vi "Q14070-Z060B - 副本.vi"() -> ()   [LabVIEW 2013]
uses:
  <vilib>/Utility/file.llb/Read From Spreadsheet File (string).vi
  <vilib>/express/express arith-compare/Formula/XNode/ExpressFormulaBlockNode.xnode
  PCI8622_32.dll
  <vilib>/printing/EasyPrintingControls.llb/contents.ctl
  <vilib>/Utility/NIReport.llb/NI_ReportGenerationCore.lvlib
  <vilib>/printing/EasyPrintingControls.llb/report_type.ctl
  <vilib>/printing/EasyPrinting.llb/Easy Print VI Panel or Documentation (path).vi
  <vilib>/Utility/NIReport.llb/NI_report.lvclass
panel:
  in  "确定按钮":bool
  out "员工ID":string
  in  "出支线工步号":dbl
  out "报警提示":string
  in  "报警工步号":dbl
  out "急停":bool
  in  "机械间隙值":dbl
  out "DeviceHandle":u32
  in  "轴向力设定次数":dbl=5.0
  in  "最小间隙(mm)":dbl=0.0005 format="%#.3f"
  out "本备料状态H":bool
  out "本测试状态H":bool
  out "本自动状态H":bool
  out "夹头松开":bool
  out "测头右位":bool
  out "测头左位":bool
  in  "测头气缸右移":bool
  in  "测头气缸左移":bool
  in  "轴向力已做次数":dbl
  out "轴向力及全行程间隙合格":bool
  out "轴向力启动":bool
  out "间隙启动":bool
  out "夹头夹紧位":bool
  in  "夹头松开":bool
  in  "夹头夹紧":bool
  out "找帽扭矩":dbl=1.0 caption="压力传感器" format="%#.2f"
  out "error out":errorcluster
  out "型号数量":i32
  out "error out 4":errorcluster
  in  "间隙设定调整次数":dbl=5.0
  out "读取产品ID":string
  out "本备料状态":bool
  out "本测试状态":bool
  out "本自动状态":bool
  out "FGCS":string
  out "KSJJ":string
  out "Z060BRFID":string
  out "轴向力Y":dbl[](array[numeric])
  out "轴向力X":dbl[](array[numeric])
  out "间隙X数组":dbl[](array[numeric])
  out "间隙Y数组":dbl[](array[numeric])
  out "error out 3":errorcluster caption="错误输出"
  out "rfid工步号":u32
  out "芯片ID":string="201209190001"
  out "rfid完成":bool
  out "rfid触发":bool
  out "本序已做":bool
  in  "回零完成":bool
  in  "电动缸回零":bool
  in  "单点间隙已调试次数":dbl
  in  "需调整角度(度)":dbl
  out "转向器中心":dbl
  out "扭矩到达":bool
  out "黄灯":bool
  out "红灯":bool
  out "基准位移":dbl caption="压力传感器" format="%#.4f"
  out "上序不合格":bool
  out "单点间隙合格":bool
  out "上序合格":bool
  out "测头机构电机":u32
  out "复位":bool
  in  "型号选择":u16(ring)=1 items=["J709", "J728", "J706"]
  in  "联线按钮":bool
  in  "工步号":u32
  in  "产品ID":string="201209190001"
  out "间隙位移(mm)":dbl caption="压力传感器" format="%#.3f"
  out "齿条推拉力(N)":dbl format="%#.2f"
  out "齿条扭矩(Nm)":dbl format="%#.2f"
  out "通讯状态":bool
  in  "员工ID":string
  out "员工姓名":string
  out "工步提示":string
  out "ADODB._Connection Out 2":refnum<k7>
  out "旋转齿条电机":u32
  out "电动缸电机":u32
  in  "停止":bool
  in  "参数加载":bool
  in  "选项卡控件":T1(tab)
  in  "180°外全行程间隙标准(mm)":dbl=0.1 format="%#.3f"
  out "扭动曲线":cluster{"Y":dbl[], "Y":dbl[]}[](graph) caption="压球涨堵头1"
  out "中间位置间隙":dbl caption="间隙值L(mm)" format="%#.3f"
  in  "中间位置最大间隙标准(mm)":dbl=0.07 format="%#.3f"
  out "右180°外全行程间隙":dbl caption="正向最大间隙L1(mm)" format="%#.3f"
  out "左180°外全行程间隙":dbl caption="正向最大间隙L1(mm)" format="%#.3f"
  out "右180°内全行程间隙":dbl caption="正向最大间隙L1(mm)" format="%#.3f"
  out "左180°内全行程间隙":dbl caption="正向最大间隙L1(mm)" format="%#.3f"
  in  "180°内全行程间隙标准(mm)":dbl=0.07 format="%#.3f"
  in  "找帽OK":bool
  out "左全行程间隙":dbl caption="正向最大间隙L1(mm)" format="%#.3f"
  out "右全行程间隙":dbl caption="正向最大间隙L1(mm)" format="%#.3f"
  out "总圈数最大值":dbl
  out "总圈数标准":dbl
  out "总行程最大值":dbl
  out "总行程标准(mm)":dbl
  out "力波动标准(N)":dbl=60.0 caption="L+Lmax(mm)" format="%#.3f"
  out "最大轴向力标准(N)":dbl=200.0 caption="L+Lmax(mm)" format="%#.3f"
  out "平均轴向力标准(N)":dbl=100.0 caption="L+Lmax(mm)" format="%#.3f"
  out "右轴向力波动(N)":dbl caption="L+Lmax(mm)" format="%#.3f"
  out "右最大轴向力(N)":dbl caption="L+Lmax(mm)" format="%#.3f"
  out "左轴向力波动(N)":dbl caption="最大位移偏离Lmax(mm)" format="%#.3f"
  out "左最大轴向力(N)":dbl caption="最大位移偏离Lmax(mm)" format="%#.3f"
  out "行程跳动曲线":cluster{"Y":dbl[], "Y":dbl[]}[](graph) caption="压球涨堵头1"
  out "右平均轴向力(N)":dbl caption="L+Lmax(mm)" format="%#.3f"
  out "左平均轴向力(N)":dbl caption="最大位移偏离Lmax(mm)" format="%#.3f"
  out "平均轴向力标准(N) max":dbl=200.0 caption="L+Lmax(mm)" format="%#.3f"
  out "总行程":dbl
  out "总圈数":dbl format="%#.2f"
  in  "不合格品":bool
  in  "扭矩停止值":dbl=16.0
  in  "齿条右极限":dbl=-70.0 caption="压力传感器" format="%#.2f"
  in  "齿条左极限":dbl=-262.0 caption="压力传感器" format="%#.2f"
  in  "齿条移动速度":dbl=5.0 caption="压力传感器" format="%#.2f"
  in  "旋转齿条轴找帽转速":dbl=5.0 caption="压力传感器" format="%#.2f"
  in  "测量点扭矩":dbl=4.0 caption="压力传感器" format="%#.2f"
  in  "旋转齿条轴测量转速":dbl caption="压力传感器" format="%#.2f"
  in  "测头机构轴后退位":dbl=30.0 caption="压力传感器" format="%#.2f"
  in  "测头机构轴待检位":dbl caption="压力传感器" format="%#.2f"
  in  "测头机构轴检测位":dbl caption="压力传感器" format="%#.2f"
  in  "测头机构轴移动速度":dbl caption="压力传感器" format="%#.2f"
  in  "全行程修正":dbl=5.5
  in  "夹头松开":bool
  in  "夹头夹紧":bool
  in  "测头气缸右移":bool
  in  "测头气缸左移":bool
  in  "支线下降":bool
  in  "支线顶升":bool
  in  "出支线":bool
  in  "进支线":bool
  in  "主线下降":bool
  in  "主线顶升":bool
  in  "下阻挡器放行":bool
  in  "上阻挡器放行":bool
  in  "测头机构轴使能":bool
  in  "测头机构轴后退":bool
  in  "测头机构轴前进":bool
  in  "电动缸速度(mm/s)":dbl=10.0 format="%#.3f"
  out "电动缸位置(mm)":dbl=10000.0 format="%#.3f"
  in  "旋转齿条轴速度(°/s)":dbl=10.0 format="%#.3f"
  out "旋转齿条轴位置(°)":dbl=10000.0 format="%#.3f"
  in  "测头机构轴速度(mm/s)":dbl=10.0 format="%#.3f"
  out "测头机构轴位置(mm)":dbl=10000.0 format="%#.3f"
  in  "旋转齿条轴右转":bool
  in  "旋转齿条轴左转":bool
  in  "旋转齿条轴使能":bool
  in  "电动缸后退":bool
  in  "电动缸使能":bool
  in  "电动缸前进":bool
  in  "齿条扭矩比例偏移":dbl=1.0 format="%#.2f"
  in  "齿条扭矩零点偏移":dbl format="%#.2f"
  in  "齿条推拉力比例偏移":dbl=1.0 format="%#.2f"
  in  "齿条推拉力零点偏移":dbl format="%#.2f"
  in  "间隙位移比例偏移":dbl=1.0 format="%#.2f"
  in  "间隙位移零点偏移":dbl format="%#.2f"
  in  "传感器参数保存":bool
  in  "参数修改":bool
  in  "参数查询":bool
  in  "参数浏览表":string[][](table)
  # "芜湖机械转向器装配线"
  # "间隙及轴向力检测"
  # "Q14070机械转向器装配线"
  # "湖北唯思凌科装备制造有限公司 设计开发 (C)2015"
  # "间隙测量结果"
  # "间隙测量判定值"
  # "≤"
  # "≤"
  # "≤"
  # "轴向力测量结果"
  # "轴向力测量标准"
  # "≥"
  # "≤"
  # "≥"
  # "≤"
  # "≤"
  # "≥"
  # "不得大于20NM"
  # "传感器校验区"
  # "关于传感器校验：\n1、传感器校验需要由具备资质的单位或部门进行校验。\n2、具备权限的用户才能够修改传感器校验参数和试验参数。\n3、修改校验参数方法：先将比例偏移置为1，修改零点偏移，使零点值与校验的传感器一致；然后根据增幅调整比例偏移。"
  # "注意：\n具备权限的用户才能够修改传感器校验参数和试验参数！"
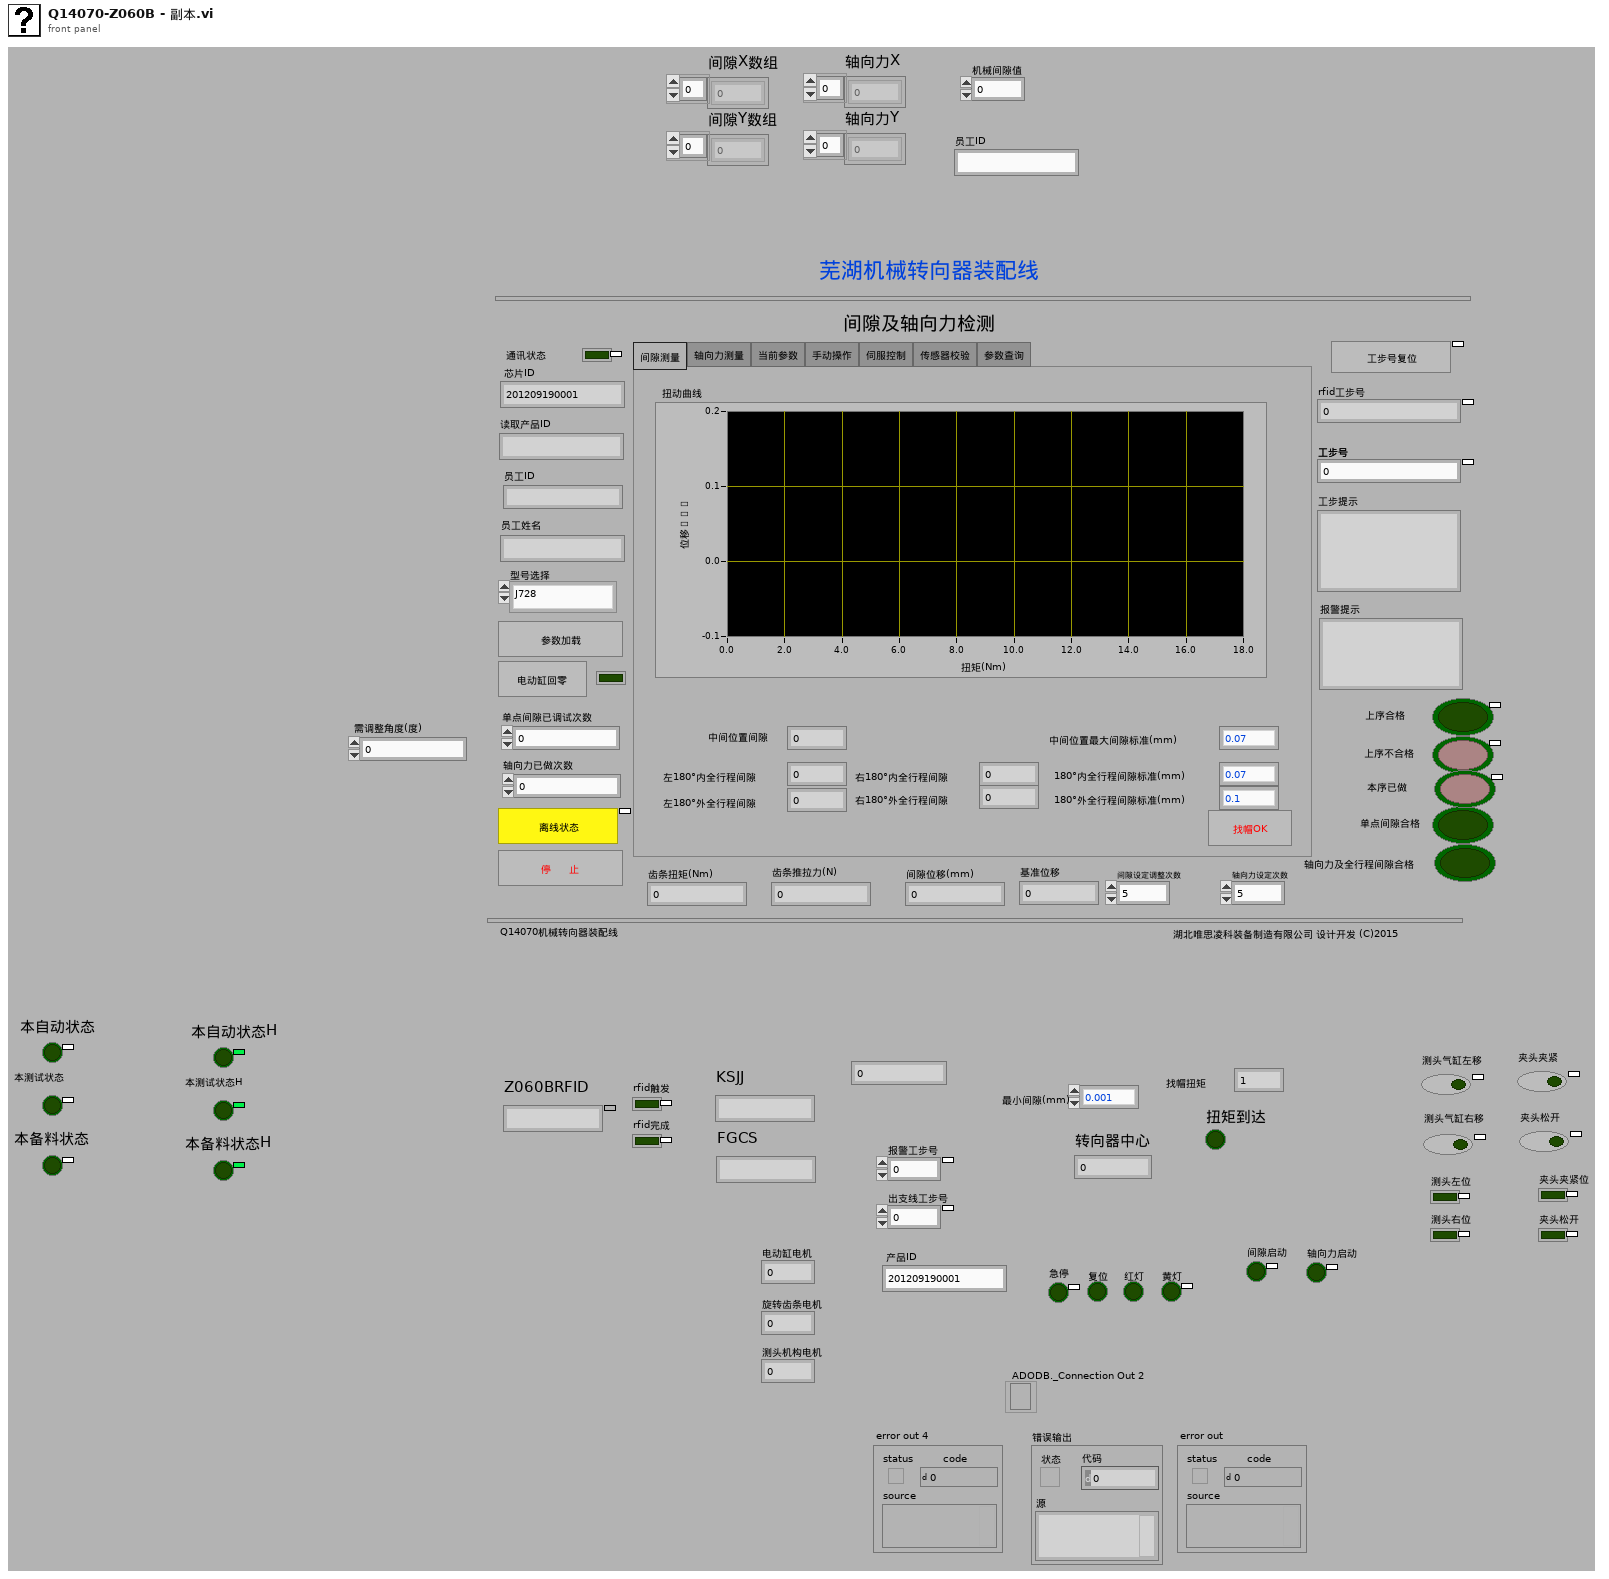
[diagram p1: front panel]
types:
  T1 = enum32{"间隙测量", "轴向力测量", "当前参数", "手动操作", "伺服控制", "传感器校验", "参数查询"}
  T2 = typedef "NI_ReportGenerationCore.lvlib/report_type.ctl" = u16
  T3 = typedef "NI_ReportGenerationCore.lvlib/contents.ctl" = u16
  T4 = typedef "imagedata.ctl" = cluster{"image type":i32, "image depth":i32, "image":u8[], "mask":u8[], "colors":u32[], "Rectangle":cluster{"left":i16, "top":i16, "right":i16, "bottom":i16}}
  T5 = enum8{"Enabled", "Disabled", "Disabled and Grayed Out"}
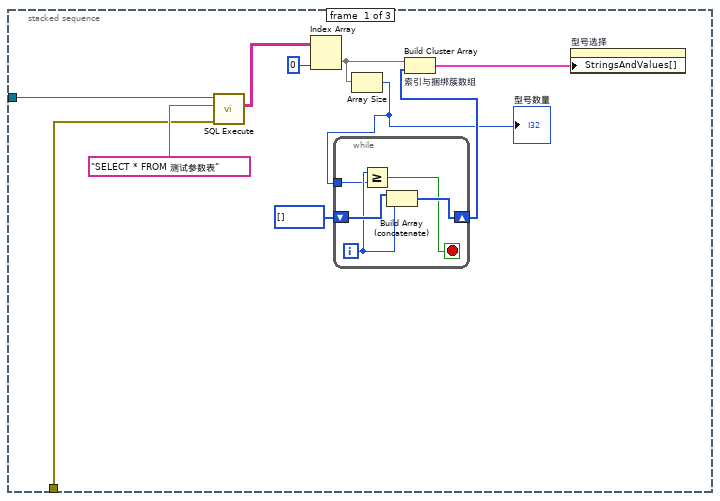
[diagram p4: hidden frame]
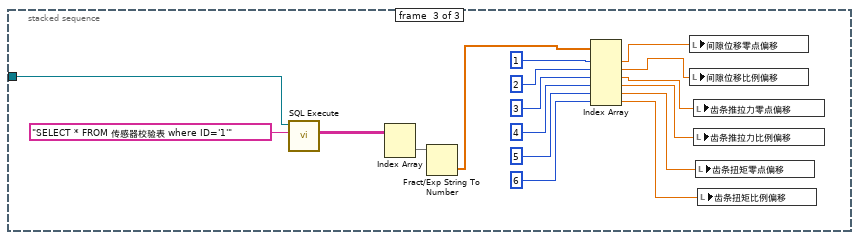
[diagram p5: hidden frame]
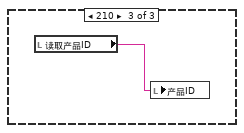
[diagram p7: hidden frame]
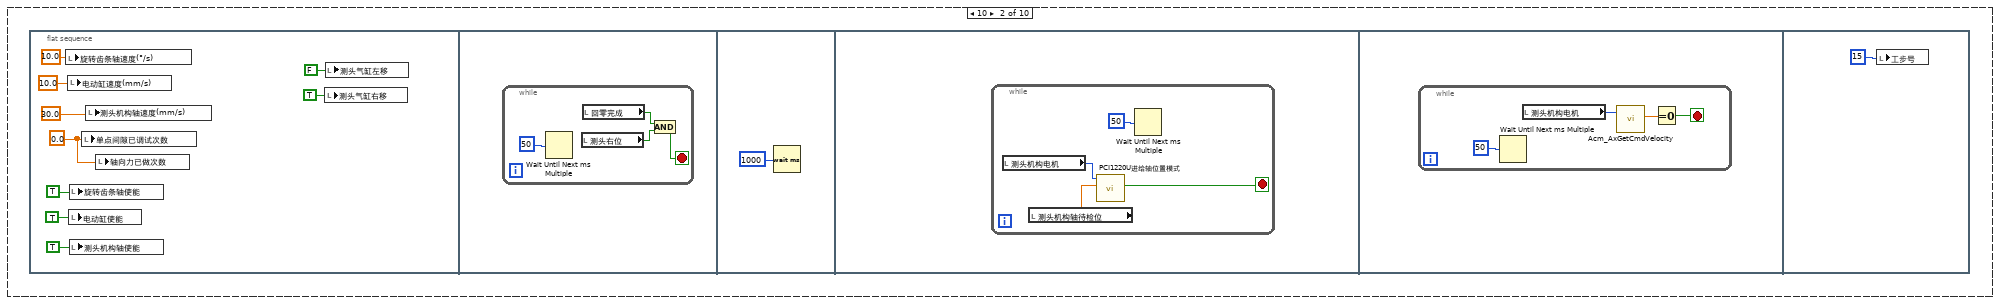
[diagram p9: hidden frame]
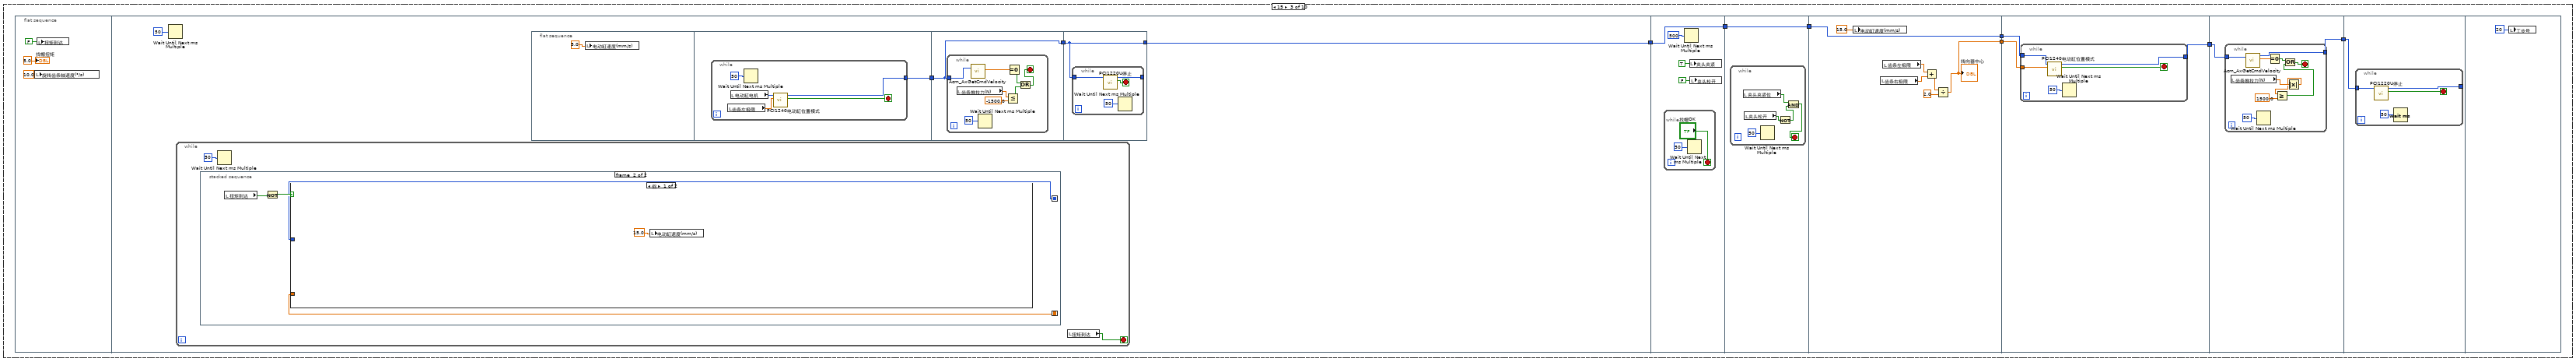
[diagram p10: hidden frame]
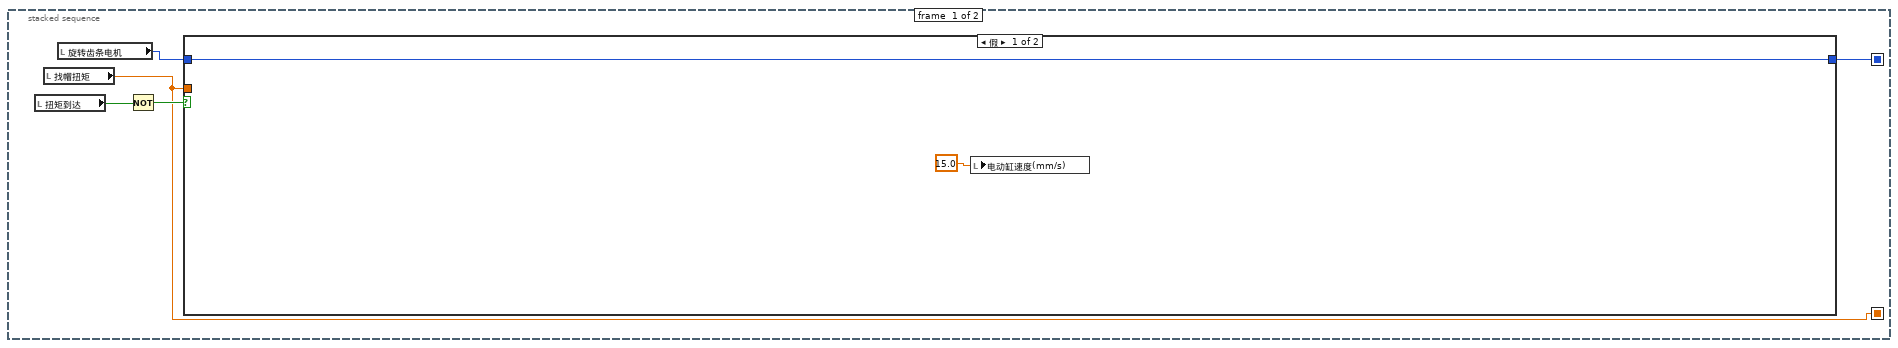
[diagram p11: hidden frame]
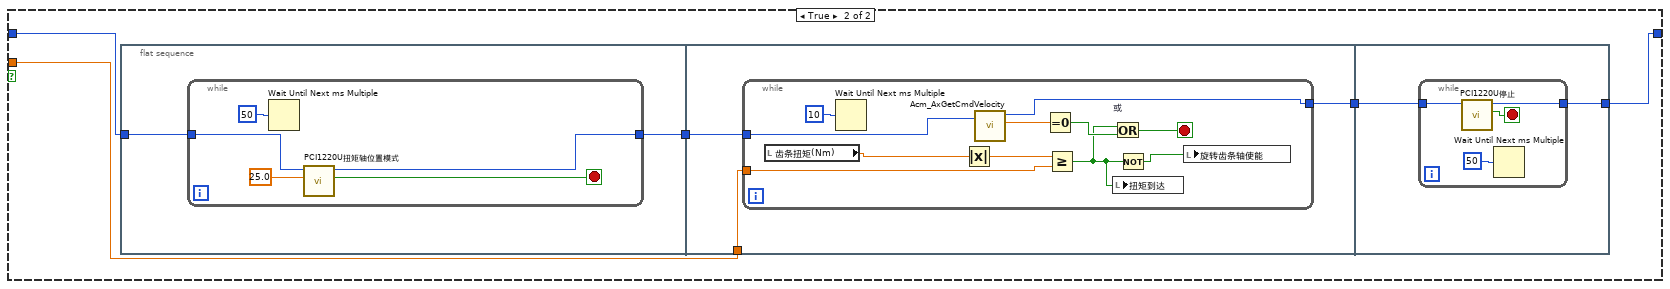
[diagram p12: hidden frame]
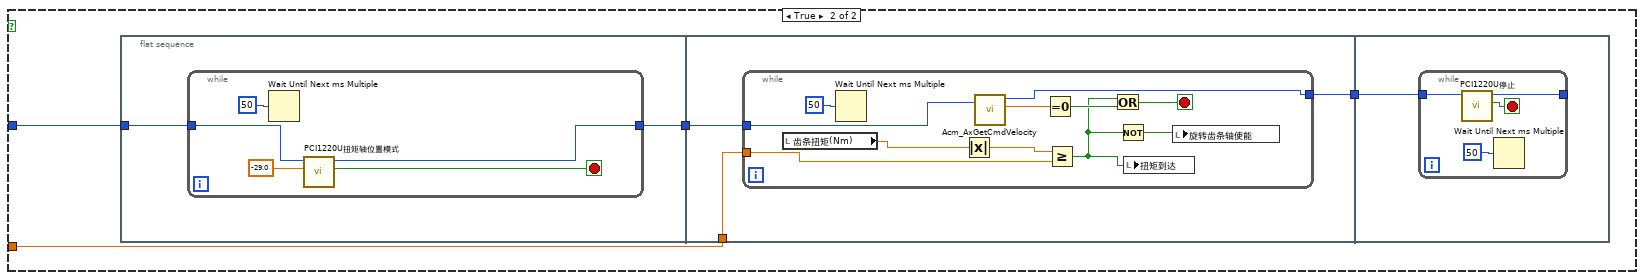
[diagram p13: hidden frame]
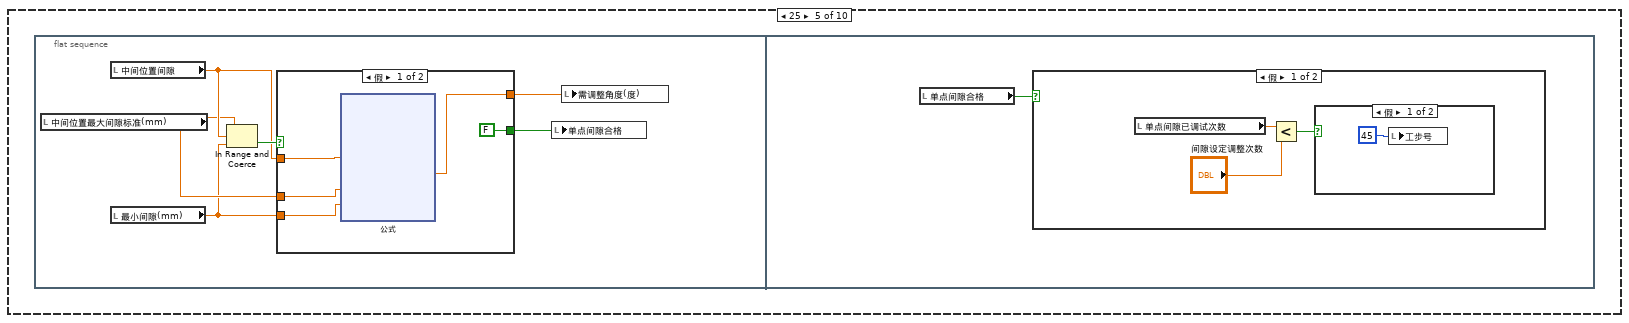
[diagram p15: hidden frame]
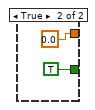
[diagram p16: hidden frame]
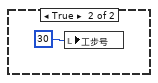
[diagram p17: hidden frame]
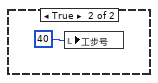
[diagram p18: hidden frame]
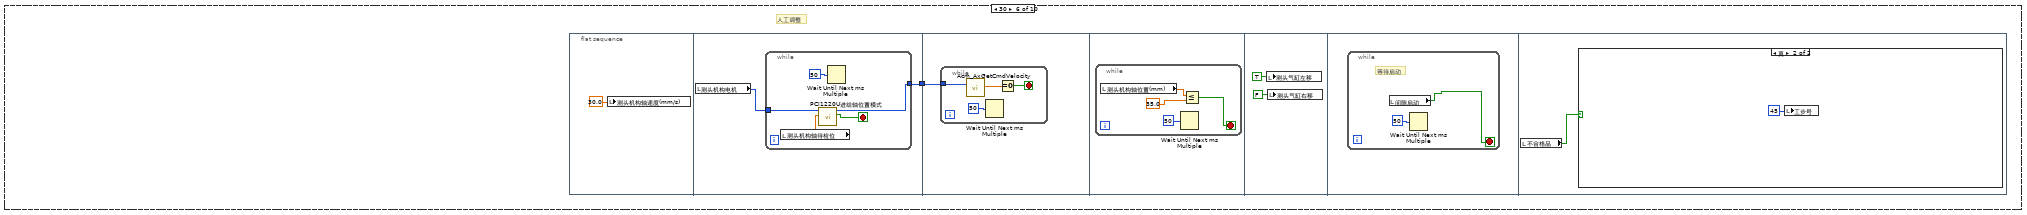
[diagram p19: hidden frame]
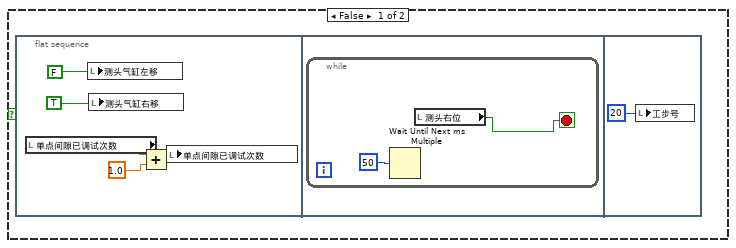
[diagram p20: hidden frame]
diagram:
  n1 = while {
    stop <- w7 stop-if-true
    n2 = local read "工步号"() -> (w5:u32)
    n3 = case shown="20" w5 {
      frame 0, Default {
      }
      frame 10 {
        n4 = flat-sequence {
          frame #0 {
            w8 = 0.0 ("已调试次数")
            n5 = local write "旋转齿条轴速度(°/s)"(10.0 ("旋转齿条轴速度(°/s)")) -> ()
            n6 = local write "电动缸速度(mm/s)"(10.0 ("电动缸速度(mm/s)")) -> ()
            n7 = local write "电动缸使能"(TRUE ("电动缸使能")) -> ()
            n8 = local write "旋转齿条轴使能"(TRUE ("旋转齿条轴使能")) -> ()
            n9 = local write "测头机构轴使能"(TRUE ("调整机构轴使能")) -> ()
            n10 = local write "单点间隙已调试次数"(w8) -> ()
            n11 = local write "测头机构轴速度(mm/s)"(30.0 ("调整机构轴速度(mm/s)")) -> ()
            n12 = local write "轴向力已做次数"(w8) -> ()
            n13 = local write "测头气缸右移"(TRUE ("测头气缸右移")) -> ()
            n14 = local write "测头气缸左移"(FALSE ("测头气缸左移")) -> ()
          }
          frame #1 {
            n15 = while {
              stop <- w17 stop-if-true
              n16 = Wait Until Next ms Multiple(millisecond multiple=u32 50 ("毫秒倍数")) -> ()  [unwired: 1 out]
              n17 = local read "测头右位"() -> (w18:bool)
              n18 = local read "回零完成"() -> (w19:bool)
              n19 = And(x=w19, y=w18) -> (x .and. y?=w17:bool)
            }
          }
          frame #2 {
            n20 = Wait (ms)(milliseconds to wait=u32 1000 ("等待时间（毫秒）")) -> ()  [unwired: 1 out]
          }
          frame #3 {
            n21 = while {
              stop <- w25 stop-if-true
              n22 = local read "测头机构电机"() -> (w23:u32)
              n23 = local read "测头机构轴待检位"() -> (w22:dbl)
              n24 = call "PCI1220U进给轴位置模式.vi"("Distance"=w22, "AxisHandle IN"=w23) -> ("AbsSuccess"=w25:bool)  [unwired: 8 in, 1 out]
              n25 = Wait Until Next ms Multiple(millisecond multiple=u32 50 ("毫秒倍数")) -> ()  [unwired: 1 out]
            }
          }
          frame #4 {
            n26 = while {
              stop <- w28 stop-if-true
              n27 = Wait Until Next ms Multiple(millisecond multiple=u32 50 ("毫秒倍数")) -> ()  [unwired: 1 out]
              n28 = local read "测头机构电机"() -> (w26:u32)
              n29 = call <userlib>:"Acm_AxGetCmdVelocity.vi"("AxisHandle"=w26) -> ("Velocity"=w29:dbl)  [unwired: 1 in, 3 out]
              n30 = Equal To 0?(x=w29) -> (x = 0?=w28:bool)
            }
          }
          frame #5 {
            n31 = local write "工步号"(u32 15 ("工步号")) -> ()
          }
        }
      }
      frame 15 {
        n32 = flat-sequence {
          tunnel: [w42] -> w34
          tunnel: w34 -> [w144]
          tunnel: [w144] -> w32
          tunnel: w32 -> [w148]
          tunnel: [w148] -> w31
          tunnel: [w159] -> w37
          tunnel: [w154] -> w36
          tunnel: w31 -> [w159]
          tunnel: w37 -> [w163]
          tunnel: w36 -> [w162]
          tunnel: [w161] -> w35
          tunnel: w35 -> [w170]
          tunnel: [w169] -> w33
          tunnel: w33 -> [w181]
          frame #0 {
            n33 = local write "旋转齿条轴速度(°/s)"(10.0 ("旋转齿条轴速度(°/s)")) -> ()
            n34 = local write "扭矩到达"(FALSE ("扭矩到达")) -> ()
            "找帽扭矩" <- 5.0 ("找帽扭矩")
          }
          frame #1 {
            n35 = Wait Until Next ms Multiple(millisecond multiple=u32 50 ("毫秒倍数")) -> ()  [unwired: 1 out]
            n36 = while {
              stop <- w45 stop-if-true
              n37 = stacked-sequence {
                seq-local: [w47 _] -> [_ w88]
                seq-local: [w51 _] -> [_ w87]
                frame #0 {
                  n38 = local read "扭矩到达"() -> (w49:bool)
                  n39 = local read "找帽扭矩"() -> (w47:dbl)
                  n40 = local read "旋转齿条电机"() -> (w48:u32)
                  n41 = Not(x=w49) -> (.not. x?=w50:bool)
                  n42 = case shown="假" w50 {
                    tunnel: [w53 w54] -> w51
                    tunnel: w48 -> [w53 w58]
                    tunnel: w47 -> [_ w56]
                    frame False {
                      n43 = local write "电动缸速度(mm/s)"(15.0 ("电动缸速度(mm/s)")) -> ()
                    }
                    frame True {
                      n44 = flat-sequence {
                        tunnel: w58 -> [w60]
                        tunnel: [w59] -> w57
                        tunnel: w57 -> [w68]
                        tunnel: w56 -> [w67]
                        tunnel: [w66] -> w55
                        tunnel: w55 -> [w81]
                        tunnel: [w80] -> w54
                        frame #0 {
                          n45 = while {
                            tunnel: [w64] -> w59
                            tunnel: w60 -> [w61]
                            stop <- w63 stop-if-true
                            n46 = Wait Until Next ms Multiple(millisecond multiple=u32 50 ("毫秒倍数")) -> ()  [unwired: 1 out]
                            n47 = call "PCI1220U扭矩轴位置模式.vi"("Distance"=25.0, "AxisHandle IN"=w61) -> ("AbsSuccess"=w63:bool, "AxisHandle OUT"=w64:u32)  [unwired: 8 in]
                          }
                        }
                        frame #1 {
                          n48 = while {
                            tunnel: w68 -> [w78]
                            tunnel: w67 -> [w73]
                            tunnel: [w72] -> w66
                            stop <- w74 stop-if-true
                            n49 = local read "齿条扭矩(Nm)"() -> (w71:dbl)
                            n50 = Wait Until Next ms Multiple(millisecond multiple=u32 10 ("毫秒倍数")) -> ()  [unwired: 1 out]
                            n51 = Absolute Value(x=w71) -> (abs(x)=w76:dbl)
                            n52 = call <userlib>:"Acm_AxGetCmdVelocity.vi"("AxisHandle"=w78) -> ("Velocity"=w77:dbl, "AxisHandle"=w72:u32)  [unwired: 1 in, 2 out]
                            n53 = Equal To 0?(x=w77) -> (x = 0?=w75:bool)
                            n54 = Greater Or Equal?(x=w76, y=w73) -> (x >= y?=w70:bool)
                            n55 = Or "或"(x=w70, y=w75) -> (x .or. y?=w74:bool)
                            n56 = local write "扭矩到达"(w70) -> ()
                            n57 = Not(x=w70) -> (.not. x?=w69:bool)
                            n58 = local write "旋转齿条轴使能"(w69) -> ()
                          }
                        }
                        frame #2 {
                          n59 = while {
                            tunnel: w81 -> [w85]
                            tunnel: [w82] -> w80
                            stop <- w84 stop-if-true
                            n60 = call "PCI1220U停止.vi"("AxisHandle IN"=w85) -> ("完成"=w84:bool, "AxisHandle OUT"=w82:u32)  [unwired: 9 in]
                            n61 = Wait Until Next ms Multiple(millisecond multiple=u32 50 ("毫秒倍数")) -> ()  [unwired: 1 out]
                          }
                        }
                      }
                    }
                  }
                }
                frame #1 {
                  n62 = local read "扭矩到达"() -> (w86:bool)
                  n63 = Not(x=w86) -> (.not. x?=w89:bool)
                  n64 = case shown="假" w89 {
                    tunnel: w87 -> [_ w94]
                    tunnel: w88 -> [_ w92]
                    frame False {
                      n65 = local write "电动缸速度(mm/s)"(15.0 ("电动缸速度(mm/s)")) -> ()
                    }
                    frame True {
                      n66 = flat-sequence {
                        tunnel: w94 -> [w95]
                        tunnel: [w96] -> w93
                        tunnel: w93 -> [w104]
                        tunnel: w92 -> [w103]
                        tunnel: [w102] -> w91
                        tunnel: w91 -> [w116]
                        frame #0 {
                          n67 = while {
                            tunnel: [w100] -> w96
                            tunnel: w95 -> [w97]
                            stop <- w99 stop-if-true
                            n68 = Wait Until Next ms Multiple(millisecond multiple=u32 50 ("毫秒倍数")) -> ()  [unwired: 1 out]
                            n69 = call "PCI1220U扭矩轴位置模式.vi"("Distance"=-29.0, "AxisHandle IN"=w97) -> ("AbsSuccess"=w99:bool, "AxisHandle OUT"=w100:u32)  [unwired: 8 in]
                          }
                        }
                        frame #1 {
                          n70 = while {
                            tunnel: w104 -> [w114]
                            tunnel: [w109] -> w102
                            tunnel: w103 -> [w108]
                            stop <- w110 stop-if-true
                            n71 = local read "齿条扭矩(Nm)"() -> (w107:dbl)
                            n72 = Wait Until Next ms Multiple(millisecond multiple=u32 50 ("毫秒倍数")) -> ()  [unwired: 1 out]
                            n73 = Absolute Value(x=w107) -> (abs(x)=w112:dbl)
                            n74 = call <userlib>:"Acm_AxGetCmdVelocity.vi"("AxisHandle"=w114) -> ("Velocity"=w113:dbl, "AxisHandle"=w109:u32)  [unwired: 1 in, 2 out]
                            n75 = Equal To 0?(x=w113) -> (x = 0?=w111:bool)
                            n76 = Greater Or Equal?(x=w112, y=w108) -> (x >= y?=w105:bool)
                            n77 = Or(x=w105, y=w111) -> (x .or. y?=w110:bool)
                            n78 = Not(x=w105) -> (.not. x?=w106:bool)
                            n79 = local write "扭矩到达"(w105) -> ()
                            n80 = local write "旋转齿条轴使能"(w106) -> ()
                          }
                        }
                        frame #2 {
                          n81 = while {
                            tunnel: w116 -> [w120]
                            tunnel: [w117] -> _
                            stop <- w119 stop-if-true
                            n82 = call "PCI1220U停止.vi"("AxisHandle IN"=w120) -> ("完成"=w119:bool, "AxisHandle OUT"=w117:u32)  [unwired: 9 in]
                            n83 = Wait Until Next ms Multiple(millisecond multiple=u32 50 ("毫秒倍数")) -> ()  [unwired: 1 out]
                          }
                        }
                      }
                    }
                  }
                }
              }
              n84 = Wait Until Next ms Multiple(millisecond multiple=u32 50 ("毫秒倍数")) -> ()  [unwired: 1 out]
              n85 = local read "扭矩到达"() -> (w45:bool)
            }
            n86 = flat-sequence {
              tunnel: [w122] -> w44
              tunnel: w44 -> [w128]
              tunnel: [w128] -> w41
              tunnel: [w137] -> w42
              tunnel: w41 -> [w137]
              frame #0 {
                n87 = local write "电动缸速度(mm/s)"(5.0 ("电动缸速度(mm/s)")) -> ()
              }
              frame #1 {
                n88 = while {
                  tunnel: [w126] -> w122
                  stop <- w125 stop-if-true
                  n89 = local read "齿条左极限"() -> (w123:dbl)
                  n90 = local read "电动缸电机"() -> (w127:u32)
                  n91 = Wait Until Next ms Multiple(millisecond multiple=u32 50 ("毫秒倍数")) -> ()  [unwired: 1 out]
                  n92 = call "PCI1240电动缸位置模式 .vi"("Distance"=w123, "AxisHandle IN"=w127) -> ("AbsSuccess"=w125:bool, "AxisHandle OUT"=w126:u32)  [unwired: 8 in]
                }
              }
              frame #2 {
                n93 = while {
                  tunnel: w128 -> [w135]
                  stop <- w132 stop-if-true
                  n94 = local read "齿条推拉力(N)"() -> (w131:dbl)
                  n95 = call <userlib>:"Acm_AxGetCmdVelocity.vi"("AxisHandle"=w135) -> ("Velocity"=w136:dbl)  [unwired: 1 in, 3 out]
                  n96 = Wait Until Next ms Multiple(millisecond multiple=u32 50 ("毫秒倍数")) -> ()  [unwired: 1 out]
                  n97 = Less Or Equal?(x=w131, y=-1500.0) -> (x <= y?=w129:bool)
                  n98 = Equal To 0?(x=w136) -> (x = 0?=w133:bool)
                  n99 = Or(x=w133, y=w129) -> (x .or. y?=w132:bool)
                }
              }
              frame #3 {
                n100 = while {
                  tunnel: w137 -> [w141]
                  tunnel: [w138] -> _
                  stop <- w140 stop-if-true
                  n101 = call "PCI1220U停止.vi"("AxisHandle IN"=w141) -> ("完成"=w140:bool, "AxisHandle OUT"=w138:u32)  [unwired: 9 in]
                  n102 = Wait Until Next ms Multiple(millisecond multiple=u32 50 ("毫秒倍数")) -> ()  [unwired: 1 out]
                }
              }
            }
          }
          frame #2 {
            n103 = while {
              stop <- "找帽OK" stop-if-true
              n104 = Wait Until Next ms Multiple(millisecond multiple=u32 50 ("毫秒倍数")) -> ()  [unwired: 1 out]
            }
            n105 = Wait Until Next ms Multiple(millisecond multiple=u32 500 ("毫秒倍数")) -> ()  [unwired: 1 out]
            n106 = local write "夹头夹紧"(TRUE ("夹头夹紧")) -> ()
            n107 = local write "夹头松开"(FALSE ("夹头松开")) -> ()
          }
          frame #3 {
            n108 = while {
              stop <- w150 stop-if-true
              n109 = local read "夹头夹紧位"() -> (w151:bool)
              n110 = local read "夹头松开"() -> (w153:bool)
              n111 = Wait Until Next ms Multiple(millisecond multiple=u32 50 ("毫秒倍数")) -> ()  [unwired: 1 out]
              n112 = Not(x=w153) -> (.not. x?=w152:bool)
              n113 = And(x=w151, y=w152) -> (x .and. y?=w150:bool)
            }
          }
          frame #4 {
            n114 = local write "电动缸速度(mm/s)"(15.0 ("电动缸轴移动速度")) -> ()
            n115 = local read "齿条右极限"() -> (w157:dbl)
            n116 = local read "齿条左极限"() -> (w158:dbl)
            n117 = Add(x=w158, y=w157) -> (x+y=w156:dbl)
            n118 = Divide(x=w156, y=2.0) -> (x/y=w154:dbl)
            "转向器中心" <- w154
          }
          frame #5 {
            n119 = while {
              tunnel: w163 -> [w168]
              tunnel: w162 -> [w167]
              tunnel: [w164] -> w161
              stop <- w166 stop-if-true
              n120 = call "PCI1240电动缸位置模式 .vi"("Distance"=w167, "AxisHandle IN"=w168) -> ("AbsSuccess"=w166:bool, "AxisHandle OUT"=w164:u32)  [unwired: 8 in]
              n121 = Wait Until Next ms Multiple(millisecond multiple=u32 50 ("毫秒倍数")) -> ()  [unwired: 1 out]
            }
          }
          frame #6 {
            n122 = while {
              tunnel: w170 -> [w180]
              tunnel: [w171] -> w169
              stop <- w172 stop-if-true
              n123 = local read "齿条推拉力(N)"() -> (w177:dbl)
              n124 = call <userlib>:"Acm_AxGetCmdVelocity.vi"("AxisHandle"=w180) -> ("Velocity"=w179:dbl, "AxisHandle"=w171:u32)  [unwired: 1 in, 2 out]
              n125 = Wait Until Next ms Multiple(millisecond multiple=u32 50 ("毫秒倍数")) -> ()  [unwired: 1 out]
              n126 = Equal To 0?(x=w179) -> (x = 0?=w174:bool)
              n127 = Absolute Value(x=w177) -> (abs(x)=w176:dbl)
              n128 = Greater Or Equal?(x=w176, y=1500.0) -> (x >= y?=w173:bool)
              n129 = Or(x=w174, y=w173) -> (x .or. y?=w172:bool)
            }
          }
          frame #7 {
            n130 = while {
              tunnel: w181 -> [w185]
              tunnel: [w184] -> _
              stop <- w183 stop-if-true
              n131 = call "PCI1220U停止.vi"("AxisHandle IN"=w185) -> ("完成"=w183:bool, "AxisHandle OUT"=w184:u32)  [unwired: 9 in]
              n132 = Wait (ms)(milliseconds to wait=u32 50 ("毫秒倍数")) -> ()  [unwired: 1 out]
            }
          }
          frame #8 {
            n133 = local write "工步号"(u32 20 ("工步号")) -> ()
          }
        }
      }
      frame 20 {
        n134 = flat-sequence {
          tunnel: [w231] -> w193
          tunnel: w193 -> [w237]
          tunnel: [w244] -> w189
          tunnel: w189 -> [w251]
          tunnel: [w251] -> w188
          tunnel: w188 -> [w259]
          tunnel: [w259] -> w187
          tunnel: w187 -> [w260]
          tunnel: [w266] -> w191
          tunnel: [w268] -> w192
          tunnel: w191 -> [w268]
          tunnel: [w270] -> w198
          tunnel: w192 -> [w270]
          tunnel: w198 -> [w277]
          tunnel: [w276] -> w197
          tunnel: [w281] -> w196
          tunnel: [w280] -> w195
          tunnel: w197 -> [w279]
          tunnel: [w279] -> w194
          tunnel: [w310] -> w201
          tunnel: [w307] -> w200
          tunnel: w196 -> [w307]
          tunnel: [w306] -> w199
          tunnel: w195 -> [w306]
          tunnel: w194 -> [w310]
          tunnel: w201 -> [w314]
          tunnel: [w313] -> w190
          tunnel: w200 -> [w311]
          tunnel: w199 -> [w312]
          tunnel: w190 -> [_]
          frame #0 {
            n135 = local write "选项卡控件"(T1."间隙测量" ("选项卡控件")) -> ()
          }
          frame #1 {
            n136 = while {
              stop <- w222 stop-if-true
              n137 = local read "夹头松开"() -> (w224:bool)
              n138 = local read "夹头夹紧位"() -> (w223:bool)
              n139 = Wait Until Next ms Multiple(millisecond multiple=u32 50 ("毫秒倍数")) -> ()  [unwired: 1 out]
              n140 = Not(x=w224) -> (.not. x?=w225:bool)
              n141 = And(x=w223, y=w225) -> (x .and. y?=w222:bool)
            }
          }
          frame #2 {
            n142 = local read "转向器中心"() -> (w227:dbl)
            n143 = local read "电动缸电机"() -> (w230:u32)
            n144 = Add(x=w227, y=0.0) -> (x+y=w229:dbl)
            n145 = while {
              tunnel: w230 -> [w236]
              tunnel: w229 -> [w235]
              tunnel: [w232] -> w231
              stop <- w234 stop-if-true
              n146 = call "PCI1240电动缸位置模式 .vi"("Distance"=w235, "AxisHandle IN"=w236) -> ("AbsSuccess"=w234:bool, "AxisHandle OUT"=w232:u32)  [unwired: 8 in]
              n147 = Wait Until Next ms Multiple(millisecond multiple=u32 50 ("毫秒倍数")) -> ()  [unwired: 1 out]
            }
          }
          frame #3 {
            n148 = while {
              tunnel: w237 -> [w241]
              stop <- w239 stop-if-true
              n149 = call <userlib>:"Acm_AxGetCmdVelocity.vi"("AxisHandle"=w241) -> ("Velocity"=w240:dbl)  [unwired: 1 in, 3 out]
              n150 = Wait Until Next ms Multiple(millisecond multiple=u32 50 ("毫秒倍数")) -> ()  [unwired: 1 out]
              n151 = Equal To 0?(x=w240) -> (x = 0?=w239:bool)
            }
          }
          frame #4 {
            n152 = local write "测头机构轴速度(mm/s)"(30.0 ("测头机构轴速度(mm/s)")) -> ()
          }
          frame #5 {
            n153 = local read "测头机构电机"() -> (w245:u32)
            n154 = local read "测头机构轴检测位"() -> (w243:dbl)
            n155 = while {
              tunnel: w245 -> [w248]
              tunnel: w243 -> [w247]
              tunnel: [w246] -> w244
              stop <- w250 stop-if-true
              n156 = Wait Until Next ms Multiple(millisecond multiple=u32 50 ("毫秒倍数")) -> ()  [unwired: 1 out]
              n157 = call "PCI1220U进给轴位置模式.vi"("Distance"=w247, "AxisHandle IN"=w248) -> ("AbsSuccess"=w250:bool, "AxisHandle OUT"=w246:u32)  [unwired: 8 in]
            }
          }
          frame #6 {
            n158 = while {
              stop <- w254 stop-if-true
              n159 = local read "测头机构轴检测位"() -> (w256:dbl)
              n160 = local read "测头机构轴位置(mm)"() -> (w253:dbl)
              n161 = Wait Until Next ms Multiple(millisecond multiple=u32 50 ("毫秒倍数")) -> ()  [unwired: 1 out]
              n162 = Subtract(x=w256, y=20.0) -> (x-y=w252:dbl)
              n163 = Greater Or Equal?(x=w253, y=w252) -> (x >= y?=w254:bool)
            }
          }
          frame #7 {
            n164 = local write "测头机构轴速度(mm/s)"(10.0 ("测头机构轴速度(mm/s)")) -> ()
          }
          frame #8 {
            n165 = while {
              tunnel: w260 -> [w264]
              stop <- w262 stop-if-true
              n166 = call <userlib>:"Acm_AxGetCmdVelocity.vi"("AxisHandle"=w264) -> ("Velocity"=w263:dbl)  [unwired: 1 in, 3 out]
              n167 = Wait Until Next ms Multiple(millisecond multiple=u32 50 ("毫秒倍数")) -> ()  [unwired: 1 out]
              n168 = Equal To 0?(x=w263) -> (x = 0?=w262:bool)
            }
          }
          frame #9 {
            n169 = local write "旋转齿条轴使能"(TRUE ("旋转齿条轴使能")) -> ()
          }
          frame #10 {
            n170 = local read "旋转齿条电机"() -> (w266:u32)
            n171 = call "PCI1220U角度置零.vi"("AxisHandle IN"=w266) -> ()  [unwired: 10 in, 1 out]
          }
          frame #11 {
            n172 = local write "旋转齿条轴速度(°/s)"(1.0 ("旋转齿条轴速度(°/s)")) -> ()
            n173 = Wait Until Next ms Multiple(millisecond multiple=u32 2000 ("毫秒倍数")) -> ()  [unwired: 1 out]
          }
          frame #12 {
            n174 = while {
              i -> [w273]
              stop <- w271 stop-if-true
              n175 = local read "间隙位移(mm)"() -> (→"基准位移":dbl)
              n176 = Wait Until Next ms Multiple(millisecond multiple=u32 500 ("毫秒倍数")) -> ()  [unwired: 1 out]
              n177 = Greater Or Equal?(x=w273, y=4) -> (x >= y?=w271:bool)
            }
          }
          frame #13 {
            n178 = call "PCI1220U运行.vi"("方向"=enum32{"Negative", "Positive"}."Negative" ("Direction"), "AxisHandle IN"=w277) -> ("AxisHandle OUT"=w276:u32)  [unwired: 9 in]
          }
          frame #14 {
            w282 = dbl[] []
            n179 = while {
              shift-right: [w293] -> w281
              shift-left: w282 -> [w295]
              shift-right: [w292] -> w280
              shift-left: w282 -> [w294]
              stop <- w285 stop-if-true
              n180 = Wait (ms)(milliseconds to wait=u32 10 ("毫秒倍数")) -> ()  [unwired: 1 out]
              n181 = local read "间隙位移(mm)"() -> (w288:dbl)
              n182 = local read "基准位移"() -> (w286:dbl)
              n183 = local read "齿条扭矩(Nm)"() -> (w289:dbl)
              n184 = Subtract(x=w288, y=w286) -> (x-y=w287:dbl)
              n185 = Absolute Value(x=w289) -> (abs(x)=w284:dbl)
              n186 = Build Array (concatenate) ("创建数组")(w294, w287) -> (w292:dbl[])
              n187 = Build Array (concatenate) ("创建数组")(w295, w284) -> (w293:dbl[])
              n188 = Greater Or Equal?(x=w284, y="扭矩停止值") -> (x >= y?=w285:bool)
              n189 = Bundle ("捆绑")(w293, w292) -> (w290:cluster{dbl[], dbl[]})  [unwired: 1 in]
              n190 = Build Array ("创建数组")(w290) -> (w291:cluster{dbl[], dbl[]}[])
              n191 = local write "扭动曲线"(w291) -> ()
            }
          }
          frame #15 {
            n192 = Absolute Value(x=w307) -> (abs(x)=w308:dbl[])
            n193 = local read "测量点扭矩"() -> (w309:dbl)
            n194 = local read "基准位移"() -> (w303:dbl)
            n195 = call "自定义插值.vi"("压力"=w309, "扭矩数组"=w308, "位移数组"=w306) -> ("扭矩值"=w304:dbl)  [unwired: 8 in]
            n196 = Array Max & Min(array=w306) -> (min value=w305:dbl)  [unwired: 3 out]
            n197 = Absolute Value(x=w305) -> (abs(x)=w302:dbl)
            n198 = Subtract(x=w303, y=w302) -> (x-y=w301:dbl)
            n199 = Add(x=w302, y=w304) -> (x+y=w299:dbl)
            n200 = local write "基准位移"(w301) -> ()
            n201 = Subtract(x=w299, y="机械间隙值") -> (x-y=w300:dbl)
            n202 = Absolute Value(x=w300) -> (abs(x)=w297:dbl)
            n203 = local write "中间位置间隙"(w297) -> ()
          }
          frame #16 {
            n204 = while {
              tunnel: w314 -> [w318]
              tunnel: [w317] -> w313
              stop <- w316 stop-if-true
              n205 = call "PCI1220U停止.vi"("AxisHandle IN"=w318) -> ("完成"=w316:bool, "AxisHandle OUT"=w317:u32)  [unwired: 9 in]
              n206 = Wait (ms)(milliseconds to wait=u32 50 ("毫秒倍数")) -> ()  [unwired: 1 out]
            }
            "间隙Y数组" <- w312
            "间隙X数组" <- w311
          }
          frame #17 {
          }
          frame #18 {
          }
          frame #19 {
          }
          frame #20 {
            n207 = local write "旋转齿条轴使能"(FALSE ("旋转齿条轴使能")) -> ()
            n208 = Wait (ms)(milliseconds to wait=u32 500 ("毫秒倍数")) -> ()  [unwired: 1 out]
          }
          frame #21 {
            n209 = local write "工步号"(u32 25 ("工步号")) -> ()
          }
        }
        n210 = disable-structure shown="禁用" {
          frame Disabled {
            n211 = while {
              tunnel: [w220] -> _
              tunnel: _ -> [w218]
              stop <- w219 stop-if-true
              n212 = Wait Until Next ms Multiple(millisecond multiple=u32 50 ("毫秒倍数")) -> ()  [unwired: 1 out]
              n213 = call "PCI1220U扭矩轴位置模式.vi"("Distance"=0.0, "AxisHandle IN"=w218) -> ("AbsSuccess"=w219:bool, "AxisHandle OUT"=w220:u32)  [unwired: 8 in]
            }
            n214 = while {
              tunnel: _ -> [w214]
              tunnel: [w206] -> _
              stop <- w207 stop-if-true
              n215 = local read "齿条扭矩(Nm)"() -> (w210:dbl)
              n216 = call <userlib>:"Acm_AxGetCmdVelocity.vi"("AxisHandle"=w214) -> ("Velocity"=w215:dbl, "AxisHandle"=w206:u32)  [unwired: 1 in, 2 out]
              n217 = Absolute Value(x=w210) -> (abs(x)=w211:dbl)
              n218 = Greater Or Equal?(x=w211, y=17.0) -> (x >= y?=w208:bool)
              n219 = Equal To 0?(x=w215) -> (x = 0?=w209:bool)
              n220 = Or(x=w209, y=w208) -> (x .or. y?=w207:bool)
              n221 = Wait Until Next ms Multiple(millisecond multiple=u32 50 ("毫秒倍数")) -> ()  [unwired: 1 out]
            }
            n222 = while {
              tunnel: _ -> [w205]
              tunnel: [w204] -> _
              stop <- w203 stop-if-true
              n223 = call "PCI1220U停止.vi"("AxisHandle IN"=w205) -> ("完成"=w203:bool, "AxisHandle OUT"=w204:u32)  [unwired: 9 in]
              n224 = Wait (ms)(milliseconds to wait=u32 50 ("毫秒倍数")) -> ()  [unwired: 1 out]
            }
          }
          frame Enabled {
          }
        }
      }
      frame 25 {
        n225 = flat-sequence {
          frame #0 {
            n226 = local read "中间位置最大间隙标准(mm)"() -> (w323:dbl)
            n227 = local read "中间位置间隙"() -> (w324:dbl)
            n228 = local read "最小间隙(mm)"() -> (w322:dbl)
            n229 = In Range and Coerce(upper limit=w323, x=w324, lower limit=w322) -> (In Range?=w327:bool)  [unwired: 1 out]
            n230 = case shown="假" w327 {
              tunnel: [FALSE ("本序合格") TRUE ("本序合格")] -> w326
              tunnel: [w332 0.0 ("需调整角度(度)")] -> w325
              tunnel: w324 -> [w330 _]
              tunnel: w323 -> [w329 _]
              tunnel: w322 -> [w328 _]
              frame False {
                n231 = xnode "公式"("X"=w330, "Xmax"=w329, "Xmin"=w328) -> ("结果"=w332:dbl)  [unwired: 1 in, 1 out]
              }
              frame True {
              }
            }
            n232 = local write "单点间隙合格"(w326) -> ()
            n233 = local write "需调整角度(度)"(w325) -> ()
          }
          frame #1 {
            n234 = local read "单点间隙合格"() -> (w347:bool)
            n235 = case shown="假" w347 {
              frame False {
                n236 = local read "单点间隙已调试次数"() -> (w350:dbl)
                n237 = Less?(x=w350, y="间隙设定调整次数") -> (x < y?=w349:bool)
                n238 = case shown="假" w349 {
                  frame False {
                    n239 = local write "工步号"(u32 45 ("变更工步号")) -> ()
                  }
                  frame True {
                    n240 = local write "工步号"(u32 30 ("变更工步号")) -> ()
                  }
                }
              }
              frame True {
                n241 = local write "工步号"(u32 40 ("变更工步号")) -> ()
              }
            }
          }
        }
      }
      frame 30 {
        # "人工调整"
        n242 = flat-sequence {
          tunnel: [w356] -> w354
          tunnel: w354 -> [w363]
          frame #0 {
            n243 = local write "测头机构轴速度(mm/s)"(30.0 ("测头机构轴速度(mm/s)")) -> ()
          }
          frame #1 {
            n244 = local read "测头机构电机"() -> (w357:u32)
            n245 = while {
              tunnel: w357 -> [w360]
              tunnel: [w359] -> w356
              stop <- w362 stop-if-true
              n246 = local read "测头机构轴待检位"() -> (w358:dbl)
              n247 = call "PCI1220U进给轴位置模式.vi"("Distance"=w358, "AxisHandle IN"=w360) -> ("AbsSuccess"=w362:bool, "AxisHandle OUT"=w359:u32)  [unwired: 8 in]
              n248 = Wait Until Next ms Multiple(millisecond multiple=u32 50 ("毫秒倍数")) -> ()  [unwired: 1 out]
            }
          }
          frame #2 {
            n249 = while {
              tunnel: w363 -> [w367]
              stop <- w365 stop-if-true
              n250 = call <userlib>:"Acm_AxGetCmdVelocity.vi"("AxisHandle"=w367) -> ("Velocity"=w366:dbl)  [unwired: 1 in, 3 out]
              n251 = Wait Until Next ms Multiple(millisecond multiple=u32 50 ("毫秒倍数")) -> ()  [unwired: 1 out]
              n252 = Equal To 0?(x=w366) -> (x = 0?=w365:bool)
            }
          }
          frame #3 {
            n253 = while {
              stop <- w369 stop-if-true
              n254 = local read "测头机构轴位置(mm)"() -> (w371:dbl)
              n255 = Wait Until Next ms Multiple(millisecond multiple=u32 50 ("毫秒倍数")) -> ()  [unwired: 1 out]
              n256 = Less Or Equal?(x=w371, y=35.0) -> (x <= y?=w369:bool)
            }
          }
          frame #4 {
            n257 = local write "测头气缸左移"(TRUE ("测头气缸左移")) -> ()
            n258 = local write "测头气缸右移"(FALSE ("测头气缸右移")) -> ()
          }
          frame #5 {
            n259 = while {
              stop <- w374 stop-if-true
              # "等待启动"
              n260 = local read "间隙启动"() -> (w374:bool)
              n261 = Wait Until Next ms Multiple(millisecond multiple=u32 50 ("毫秒倍数")) -> ()  [unwired: 1 out]
            }
          }
          frame #6 {
            n262 = local read "不合格品"() -> (w376:bool)
            n263 = case shown="真" w376 {
              frame False {
                n264 = flat-sequence {
                  frame #0 {
                    n265 = local read "单点间隙已调试次数"() -> (w379:dbl)
                    n266 = local write "测头气缸左移"(FALSE ("测头气缸左移")) -> ()
                    n267 = local write "测头气缸右移"(TRUE ("测头气缸左移")) -> ()
                    n268 = Add(x=w379, y=1.0 ("已调试次数")) -> (x+y=w381:dbl)
                    n269 = local write "单点间隙已调试次数"(w381) -> ()
                  }
                  frame #1 {
                    n270 = while {
                      stop <- w382 stop-if-true
                      n271 = Wait Until Next ms Multiple(millisecond multiple=u32 50 ("毫秒倍数")) -> ()  [unwired: 1 out]
                      n272 = local read "测头右位"() -> (w382:bool)
                    }
                  }
                  frame #2 {
                    n273 = local write "工步号"(u32 20 ("工步号")) -> ()
                  }
                }
              }
              frame True {
                n274 = local write "工步号"(u32 45 ("工步号")) -> ()
              }
            }
          }
        }
      }
      frame 40 {
        n275 = flat-sequence {
          tunnel: [w482] -> w478
          tunnel: w478 -> [w484]
          tunnel: [w483] -> w476
          tunnel: w476 -> [w490]
          tunnel: [w490] -> w455
          tunnel: w455 -> [w499]
          tunnel: [w499] -> w454
          tunnel: w454 -> [w506]
          tunnel: [w506] -> w475
          tunnel: w475 -> [w508]
          tunnel: [w509] -> w453
          tunnel: [w507] -> w452
          tunnel: [w521] -> w468
          tunnel: [w520] -> w466
          tunnel: [w519] -> w464
          tunnel: w453 -> [w518]
          tunnel: [w518] -> w462
          tunnel: [w516] -> w458
          tunnel: w452 -> [w515]
          tunnel: w468 -> [w563]
          tunnel: [w563] -> w467
          tunnel: w466 -> [w570]
          tunnel: [w570] -> w465
          tunnel: w464 -> [w566]
          tunnel: [w566] -> w463
          tunnel: w462 -> [w569]
          tunnel: [w569] -> w461
          tunnel: [w565] -> w459
          tunnel: w458 -> [w565]
          tunnel: [w567] -> w456
          tunnel: [w555] -> w440
          tunnel: [w564] -> w439
          tunnel: [w556] -> w437
          tunnel: [w562] -> w432
          tunnel: w467 -> [w591]
          tunnel: [w591] -> w474
          tunnel: w465 -> [w590]
          tunnel: [w590] -> w473
          tunnel: w463 -> [w589]
          tunnel: [w589] -> w472
          tunnel: w461 -> [w588]
          tunnel: [w588] -> w470
          tunnel: [w587] -> w460
          tunnel: w459 -> [w587]
          tunnel: [w586] -> w457
          tunnel: w456 -> [w586]
          tunnel: w440 -> [w582]
          tunnel: w439 -> [w585]
          tunnel: w437 -> [w583]
          tunnel: w432 -> [w584]
          tunnel: [w584] -> w431
          tunnel: [w581] -> w416
          tunnel: [w576] -> w409
          tunnel: [w575] -> w408
          tunnel: [w609] -> w451
          tunnel: [w608] -> w450
          tunnel: w474 -> [w607]
          tunnel: w473 -> [w606]
          tunnel: w472 -> [w605]
          tunnel: [w604] -> w448
          tunnel: w470 -> [w603]
          tunnel: [w603] -> w446
          tunnel: w460 -> [w602]
          tunnel: w457 -> [w600]
          tunnel: [w601] -> w444
          tunnel: [w600] -> w442
          tunnel: w431 -> [w599]
          tunnel: [w599] -> w430
          tunnel: w416 -> [w598]
          tunnel: [w598] -> w414
          tunnel: w409 -> [w596]
          tunnel: w408 -> [w597]
          tunnel: [w597] -> w405
          tunnel: [w596] -> w404
          tunnel: w451 -> [w647]
          tunnel: w450 -> [w655]
          tunnel: [w655] -> w449
          tunnel: w448 -> [w651]
          tunnel: [w651] -> w447
          tunnel: w446 -> [w654]
          tunnel: [w654] -> w445
          tunnel: w444 -> [w653]
          tunnel: [w653] -> w443
          tunnel: w442 -> [w652]
          tunnel: [w652] -> w441
          tunnel: w430 -> [w648]
          tunnel: [w648] -> w429
          tunnel: [w647] -> w428
          tunnel: [w646] -> w427
          tunnel: [w645] -> w426
          tunnel: [w644] -> w415
          tunnel: w414 -> [w644]
          tunnel: w405 -> [w642]
          tunnel: w404 -> [w643]
          tunnel: [w643] -> w403
          tunnel: [w642] -> w402
          tunnel: w449 -> [w683]
          tunnel: [w698] -> w477
          tunnel: w447 -> [w698]
          tunnel: [w697] -> w469
          tunnel: w445 -> [w697]
          tunnel: w443 -> [w696]
          tunnel: w441 -> [w695]
          tunnel: [w693] -> w438
          tunnel: w429 -> [w692]
          tunnel: w428 -> [w691]
          tunnel: w427 -> [w689]
          tunnel: w426 -> [w688]
          tunnel: [w686] -> w425
          tunnel: [w685] -> w424
          tunnel: [w684] -> w423
          tunnel: w415 -> [w679]
          tunnel: [w679] -> w412
          tunnel: [w678] -> w407
          tunnel: [w677] -> w406
          tunnel: w403 -> [w676]
          tunnel: w402 -> [w675]
          tunnel: [w676] -> w401
          tunnel: [w675] -> w400
          tunnel: [w674] -> w395
          tunnel: [w673] -> w393
          tunnel: [w670] -> w390
          tunnel: [w665] -> w388
          tunnel: [w660] -> w386
          tunnel: w477 -> [w726]
          tunnel: [w726] -> w422
          tunnel: w469 -> [_]
          tunnel: [w722] -> w420
          tunnel: w438 -> [w724]
          tunnel: [w721] -> w418
          tunnel: w425 -> [w720]
          tunnel: w424 -> [w719]
          tunnel: w423 -> [w718]
          tunnel: [w717] -> w413
          tunnel: w412 -> [w717]
          tunnel: [w716] -> w411
          tunnel: [w715] -> w410
          tunnel: w407 -> [w714]
          tunnel: w406 -> [w713]
          tunnel: w401 -> [w708]
          tunnel: w400 -> [w707]
          tunnel: [w708] -> w399
          tunnel: [w707] -> w398
          tunnel: [w706] -> w397
          tunnel: [w705] -> w396
          tunnel: w395 -> [w705]
          tunnel: [w704] -> w394
          tunnel: w393 -> [w704]
          tunnel: [w703] -> w392
          tunnel: [w702] -> w391
          tunnel: w390 -> [w701]
          tunnel: [w700] -> w389
          tunnel: w388 -> [w700]
          tunnel: [w699] -> w387
          tunnel: w386 -> [w699]
          tunnel: w422 -> [w744]
          tunnel: [w744] -> w421
          tunnel: w420 -> [w743]
          tunnel: [w743] -> w419
          tunnel: w418 -> [w742]
          tunnel: [w742] -> w417
          tunnel: w413 -> [w738]
          tunnel: w411 -> [w736]
          tunnel: w410 -> [w735]
          tunnel: w399 -> [w739]
          tunnel: w398 -> [w737]
          tunnel: w397 -> [w734]
          tunnel: w396 -> [w733]
          tunnel: w394 -> [w732]
          tunnel: w392 -> [w731]
          tunnel: w391 -> [w730]
          tunnel: w389 -> [w728]
          tunnel: w387 -> [w727]
          tunnel: w421 -> [w748]
          tunnel: [w747] -> w471
          tunnel: w419 -> [w746]
          tunnel: w417 -> [w745]
          tunnel: [w745] -> w434
          tunnel: w471 -> [w755]
          tunnel: [w755] -> w436
          tunnel: w434 -> [w754]
          tunnel: [w754] -> w433
          tunnel: w436 -> [w762]
          tunnel: [w761] -> w435
          tunnel: w433 -> [w760]
          tunnel: w435 -> [w768]
          frame #0 {
            n276 = local write "选项卡控件"(T1."轴向力测量" ("选项卡控件")) -> ()
          }
          frame #1 {
            n277 = local write "电动缸速度(mm/s)"(15.0 ("电动缸速度(mm/s)")) -> ()
            n278 = local write "单点间隙已调试次数"(0.0 ("单点间隙已调试次数")) -> ()
            n279 = local read "电动缸电机"() -> (w482:u32)
          }
          frame #2 {
            n280 = while {
              tunnel: w484 -> [w489]
              tunnel: [w488] -> w483
              stop <- w487 stop-if-true
              n281 = local read "齿条左极限"() -> (w485:dbl)
              n282 = Wait (ms)(milliseconds to wait=u32 50 ("毫秒倍数")) -> ()  [unwired: 1 out]
              n283 = call "PCI1240电动缸位置模式 .vi"("Distance"=w485, "AxisHandle IN"=w489) -> ("AbsSuccess"=w487:bool, "AxisHandle OUT"=w488:u32)  [unwired: 8 in]
            }
          }
          frame #3 {
            n284 = while {
              tunnel: w490 -> [w498]
              stop <- w491 stop-if-true
              n285 = local read "齿条推拉力(N)"() -> (w495:dbl)
              n286 = call <userlib>:"Acm_AxGetCmdVelocity.vi"("AxisHandle"=w498) -> ("Velocity"=w497:dbl)  [unwired: 1 in, 3 out]
              n287 = Wait Until Next ms Multiple(millisecond multiple=u32 50 ("毫秒倍数")) -> ()  [unwired: 1 out]
              n288 = Equal To 0?(x=w497) -> (x = 0?=w493:bool)
              n289 = Less Or Equal?(x=w495, y=-1000.0) -> (x <= y?=w492:bool)
              n290 = Or ("或")(x=w493, y=w492) -> (x .or. y?=w491:bool)
            }
          }
          frame #4 {
            n291 = while {
              tunnel: w499 -> [w503]
              tunnel: [w502] -> _
              stop <- w501 stop-if-true
              n292 = call "PCI1220U停止.vi"("AxisHandle IN"=w503) -> ("完成"=w501:bool, "AxisHandle OUT"=w502:u32)  [unwired: 9 in]
              n293 = Wait (ms)(milliseconds to wait=u32 50 ("毫秒倍数")) -> ()  [unwired: 1 out]
            }
          }
          frame #5 {
            n294 = Wait Until Next ms Multiple(millisecond multiple=u32 50 ("毫秒倍数")) -> ()  [unwired: 1 out]
            n295 = local write "电动缸速度(mm/s)"(15.0 ("电动缸速度(mm/s)")) -> ()
          }
          frame #6 {
            n296 = while {
              tunnel: w508 -> [w514]
              tunnel: [w511] -> w507
              stop <- w512 stop-if-true
              n297 = local read "齿条右极限"() -> (w510:dbl)
              n298 = Wait Until Next ms Multiple(millisecond multiple=u32 50 ("毫秒倍数")) -> ()  [unwired: 1 out]
              n299 = call "PCI1240电动缸位置模式 .vi"("Distance"=w510, "AxisHandle IN"=w514) -> ("AbsSuccess"=w512:bool, "AxisHandle OUT"=w511:u32)  [unwired: 8 in]
            }
            n300 = local read "转向器中心"() -> (w509:dbl)
          }
          frame #7 {
            w517 = dbl[] []
            n301 = while {
              shift-right: [w541] -> w520
              shift-left: w517 -> [w552]
              shift-right: [w550] -> w521
              shift-left: w517 -> [w551]
              tunnel: w515 -> [w546]
              tunnel: [w546] -> w519
              tunnel: w518 -> [w544]
              shift-right: [w540] -> w516
              shift-left: w517 -> [w542]
              stop <- w534 stop-if-true
              n302 = local read "中间位置间隙"() -> (w531:dbl)
              n303 = local read "基准位移"() -> (w547:dbl)
              n304 = local read "间隙位移(mm)"() -> (w530:dbl)
              n305 = call <userlib>:"Acm_AxGetCmdVelocity.vi"("AxisHandle"=w546) -> ("Velocity"=w539:dbl)  [unwired: 1 in, 3 out]
              n306 = Wait (ms)(milliseconds to wait=u32 50 ("毫秒倍数")) -> ()  [unwired: 1 out]
              n307 = local read "齿条推拉力(N)"() -> (w537:dbl)
              n308 = call "PCI1240电动缸读取位置.vi"("AxisHandle IN"=w546) -> ("位置"=w545:dbl)  [unwired: 9 in, 1 out]
              n309 = Subtract(x=w530, y=w547) -> (x-y=w533:dbl)
              n310 = Subtract(x=w545, y=w544) -> (x-y=w524:dbl)
              n311 = Add(x=w533, y=w531) -> (x+y=w532:dbl)
              n312 = Multiply(x=w524, y=1.12) -> (x*y=w522:dbl)
              n313 = Build Array (concatenate) ("创建数组")(w551, w532) -> (w550:dbl[])
              n314 = Build Array (concatenate) ("创建数组")(w552, w522) -> (w541:dbl[])
              n315 = Build Array (concatenate) ("创建数组")(w542, w537) -> (w540:dbl[])
              n316 = Greater Or Equal?(x=w537, y=1000.0) -> (x >= y?=w535:bool)
              n317 = Less Or Equal?(x=w530, y=-1.0) -> (x <= y?=w529:bool)
              n318 = Greater Or Equal?(x=w530, y=4.0) -> (x >= y?=w528:bool)
              n319 = Equal To 0?(x=w539) -> (x = 0?=w536:bool)
              n320 = Or(x=w528, y=w529) -> (x .or. y?=w527:bool)
              n321 = Bundle ("捆绑")(w541, w550) -> (w548:cluster{dbl[], dbl[]})  [unwired: 1 in]
              n322 = Or(x=w536, y=w535) -> (x .or. y?=w534:bool)
              n323 = Bundle ("捆绑")(w541, w540) -> (w543:cluster{dbl[], dbl[]})  [unwired: 1 in]
              n324 = property on="间隙位移(mm)" class="DigNum (严格)"("Blinking"=w527) -> ()  [unwired: 2 in, 2 out]
              n325 = Build Array ("创建数组")(w548, w543) -> (w549:cluster{dbl[], dbl[]}[])
              n326 = local write "行程跳动曲线"(w549) -> ()
            }
          }
          frame #8 {
            n327 = while {
              tunnel: w566 -> [w574]
              tunnel: [w573] -> _
              stop <- w572 stop-if-true
              n328 = call "PCI1220U停止.vi"("AxisHandle IN"=w574) -> ("完成"=w572:bool, "AxisHandle OUT"=w573:u32)  [unwired: 9 in]
              n329 = Wait (ms)(milliseconds to wait=u32 50 ("毫秒倍数")) -> ()  [unwired: 1 out]
            }
            n330 = Array Size(array=w565) -> (size(s)=w567:i32)
            n331 = Array Size(array=w563) -> (size(s)=w562:i32)
            n332 = Wait Until Next ms Multiple(millisecond multiple=u32 500 ("毫秒倍数")) -> ()  [unwired: 1 out]
            n333 = call "功能计算.vi"("扭矩数组"=w565) -> ("扭差"=w556:dbl, "平均扭矩"=w564:dbl, "峰值扭矩"=w555:dbl)  [unwired: 7 in, 1 out]
            "左轴向力波动(N)" <- w556
            "左最大轴向力(N)" <- w555
            n334 = call "间隙计算.vi"("扭矩数组"=w563) -> ("峰值间隙1"=w561:dbl, "峰值间隙2"=w560:dbl)  [unwired: 6 in, 3 out]
            n335 = local read "180°内全行程间隙标准(mm)"() -> (w559:dbl)
            n336 = local read "180°外全行程间隙标准(mm)"() -> (w554:dbl)
            n337 = local write "左平均轴向力(N)"(w564) -> ()
            n338 = local write "左180°外全行程间隙"(w560) -> ()
            n339 = local write "左180°内全行程间隙"(w561) -> ()
            n340 = Greater?(x=w561, y=w559) -> (0:w558:bool)
            n341 = Greater?(x=w560, y=w554) -> (0:w557:bool)
            n342 = property on="左180°内全行程间隙" class="DigNum (严格)"("Blinking"=w558) -> ()  [unwired: 2 in, 2 out]
            n343 = property on="左180°外全行程间隙" class="DigNum (严格)"("Blinking"=w557) -> ()  [unwired: 2 in, 2 out]
          }
          frame #9 {
            n344 = local read "最大轴向力标准(N)"() -> (w580:dbl)
            n345 = local read "平均轴向力标准(N)"() -> (w579:dbl)
            n346 = while {
              tunnel: w589 -> [w595]
              tunnel: w588 -> [_]
              stop <- w594 stop-if-true
              n347 = Wait Until Next ms Multiple(millisecond multiple=u32 50 ("毫秒倍数")) -> ()  [unwired: 1 out]
              n348 = local read "齿条左极限"() -> (w592:dbl)
              n349 = call "PCI1240电动缸位置模式 .vi"("Distance"=w592, "AxisHandle IN"=w595) -> ("AbsSuccess"=w594:bool)  [unwired: 8 in, 1 out]
            }
            n350 = local read "平均轴向力标准(N) max"() -> (w578:dbl)
            n351 = local read "力波动标准(N)"() -> (w577:dbl)
            n352 = call "判断.vi"("y 3"=w577, "y 2-2"=w578, "y 2-1"=w579, "y"=w580, "x 3"=w583, "x 2"=w585, "x"=w582) -> ("非x? 3"=w575:bool, "非x? 2"=w581:bool, "非x?"=w576:bool)  [unwired: 2 in]
            n353 = property on="左最大轴向力(N)" class="DigNum (严格)"("Blinking"=w576) -> ()  [unwired: 2 in, 2 out]
            n354 = property on="左平均轴向力(N)" class="DigNum (严格)"("Blinking"=w581) -> ()  [unwired: 2 in, 2 out]
            n355 = property on="左轴向力波动(N)" class="DigNum (严格)"("Blinking"=w575) -> ()  [unwired: 2 in, 2 out]
          }
          frame #10 {
            n356 = while {
              shift-right: [w630] -> w608
              shift-left: w606 -> [w640]
              shift-right: [w638] -> w609
              shift-left: w607 -> [w639]
              tunnel: w605 -> [w633]
              tunnel: [w633] -> w604
              tunnel: w603 -> [w631]
              shift-right: [w627] -> w601
              shift-left: w602 -> [w628]
              stop <- w622 stop-if-true
              n357 = call <userlib>:"Acm_AxGetCmdVelocity.vi"("AxisHandle"=w633) -> ("Velocity"=w620:dbl)  [unwired: 1 in, 3 out]
              n358 = local read "间隙位移(mm)"() -> (w614:dbl)
              n359 = local read "基准位移"() -> (w634:dbl)
              n360 = Wait (ms)(milliseconds to wait=u32 50 ("毫秒倍数")) -> ()  [unwired: 1 out]
              n361 = local read "中间位置间隙"() -> (w619:dbl)
              n362 = local read "齿条推拉力(N)"() -> (w626:dbl)
              n363 = call "PCI1240电动缸读取位置.vi"("AxisHandle IN"=w633) -> ("位置"=w632:dbl)  [unwired: 9 in, 1 out]
              n364 = Subtract(x=w614, y=w634) -> (x-y=w635:dbl)
              n365 = Subtract(x=w632, y=w631) -> (x-y=w612:dbl)
              n366 = Add(x=w635, y=w619) -> (x+y=w621:dbl)
              n367 = Multiply(x=w612, y=1.12) -> (x*y=w610:dbl)
              n368 = Build Array (concatenate) ("创建数组")(w640, w610) -> (w630:dbl[])
              n369 = Less Or Equal?(x=w626, y=-1000.0) -> (x <= y?=w623:bool)
              n370 = Build Array (concatenate) ("创建数组")(w628, w626) -> (w627:dbl[])
              n371 = Equal To 0?(x=w620) -> (x = 0?=w624:bool)
              n372 = Build Array (concatenate) ("创建数组")(w639, w621) -> (w638:dbl[])
              n373 = Bundle ("捆绑")(w630, w627) -> (w629:cluster{dbl[], dbl[]})  [unwired: 1 in]
              n374 = Or(x=w624, y=w623) -> (x .or. y?=w622:bool)
              n375 = Bundle ("捆绑")(w630, w638) -> (w636:cluster{dbl[], dbl[]})  [unwired: 1 in]
              n376 = Build Array ("创建数组")(w636, w629) -> (w637:cluster{dbl[], dbl[]}[])
              n377 = Less Or Equal?(x=w614, y=-1.0) -> (x <= y?=w618:bool)
              n378 = Greater Or Equal?(x=w614, y=4.0) -> (x >= y?=w617:bool)
              n379 = local write "行程跳动曲线"(w637) -> ()
              n380 = Or(x=w617, y=w618) -> (x .or. y?=w613:bool)
              n381 = property on="间隙位移(mm)" class="DigNum (严格)"("Blinking"=w613) -> ()  [unwired: 2 in, 2 out]
            }
          }
          frame #11 {
            n382 = while {
              tunnel: w651 -> [w659]
              tunnel: [w658] -> _
              stop <- w657 stop-if-true
              n383 = call "PCI1220U停止.vi"("AxisHandle IN"=w659) -> ("完成"=w657:bool, "AxisHandle OUT"=w658:u32)  [unwired: 9 in]
              n384 = Wait (ms)(milliseconds to wait=u32 50 ("毫秒倍数")) -> ()  [unwired: 1 out]
            }
            n385 = Array Max & Min(array=w647) -> (max value=w650:dbl, min value=w649:dbl)  [unwired: 2 out]
            n386 = Absolute Value(x=w650) -> (abs(x)=w646:dbl)
            n387 = Absolute Value(x=w649) -> (abs(x)=w645:dbl)
            n388 = local write "左全行程间隙"(w646) -> ()
            n389 = local write "右全行程间隙"(w645) -> ()
          }
          frame #12 {
            n390 = local read "180°内全行程间隙标准(mm)"() -> (w687:dbl)
            n391 = Split 1D Array(array=w696, index=w695) -> (second subarray=w694:dbl[])  [unwired: 1 out]
            n392 = Array Max & Min(array=w683) -> (max value=w682:dbl, min value=w681:dbl)  [unwired: 2 out]
            n393 = local read "全行程修正"() -> (w671:dbl)
            n394 = local read "总圈数标准"() -> (w663:dbl)
            n395 = local read "总圈数最大值"() -> (w664:dbl)
            n396 = Subtract(x=w682, y=w681) -> (x-y=w672:dbl)
            n397 = call "功能计算.vi"("扭矩数组"=w694) -> ("扭差"=w677:dbl, "平均扭矩"=w693:dbl, "峰值扭矩"=w678:dbl)  [unwired: 7 in, 1 out]
            n398 = Subtract(x=w672, y=w671) -> (x-y=w669:dbl)
            n399 = Split 1D Array(array=w691, index=w692) -> (second subarray=w690:dbl[])  [unwired: 1 out]
            n400 = Greater?(x=w689, y=w687) -> (0:w674:bool)
            n401 = Greater?(x=w688, y=w687) -> (0:w673:bool)
            n402 = local write "右最大轴向力(N)"(w678) -> ()
            n403 = call "间隙计算.vi"("扭矩数组"=w690) -> ("峰值间隙1"=w685:dbl, "峰值间隙2"=w684:dbl)  [unwired: 6 in, 3 out]
            n404 = Divide(x=w669, y=46.996) -> (x/y=w662:dbl)
            n405 = In Range and Coerce(upper limit=w664, x=w662, lower limit=w663) -> (In Range?=w661:bool)  [unwired: 1 out]
            n406 = Not(x=w661) -> (.not. x?=w660:bool)
            n407 = property on="总圈数" class="DigNum (严格)"("Blinking"=w660) -> ()  [unwired: 2 in, 2 out]
            n408 = property on="左全行程间隙" class="DigNum (严格)"("Blinking"=w674) -> ()  [unwired: 2 in, 2 out]
            n409 = property on="右全行程间隙" class="DigNum (严格)"("Blinking"=w673) -> ()  [unwired: 2 in, 2 out]
            n410 = local write "右平均轴向力(N)"(w693) -> ()
            n411 = local write "右轴向力波动(N)"(w677) -> ()
            n412 = local write "总圈数"(w662) -> ()
            n413 = local read "180°内全行程间隙标准(mm)"() -> (w686:dbl)
            n414 = local read "总行程标准(mm)"() -> (w667:dbl)
            n415 = local read "总行程最大值"() -> (w668:dbl)
            n416 = In Range and Coerce(upper limit=w668, x=w669, lower limit=w667) -> (In Range?=w666:bool)  [unwired: 1 out]
            n417 = local write "右180°外全行程间隙"(w684) -> ()
            n418 = local write "右180°内全行程间隙"(w685) -> ()
            n419 = local read "180°外全行程间隙标准(mm)"() -> (w670:dbl)
            n420 = Not(x=w666) -> (.not. x?=w665:bool)
            n421 = local write "总行程"(w669) -> ()
            n422 = property on="总行程" class="DigNum (严格)"("Blinking"=w665) -> ()  [unwired: 2 in, 2 out]
            "轴向力X" <- w683
            "轴向力Y" <- w696
          }
          frame #13 {
            n423 = local read "最大轴向力标准(N)"() -> (w712:dbl)
            n424 = local read "平均轴向力标准(N)"() -> (w711:dbl)
            n425 = local read "平均轴向力标准(N) max"() -> (w710:dbl)
            n426 = Greater?(x=w719, y=w720) -> (0:w703:bool)
            n427 = Greater?(x=w718, y=w701) -> (0:w702:bool)
            n428 = local write "电动缸速度(mm/s)"(15.0 ("电动缸速度(mm/s)")) -> ()
            n429 = local read "转向器中心"() -> (w721:dbl)
            n430 = local read "力波动标准(N)"() -> (w709:dbl)
            n431 = call "判断.vi"("y 3"=w709, "y 2-2"=w710, "y 2-1"=w711, "y"=w712, "x 3"=w713, "x 2"=w724, "x"=w714) -> ("非x? 3"=w706:bool, "非x? 2"=w715:bool, "非x?"=w716:bool)  [unwired: 2 in]
            n432 = property on="右180°内全行程间隙" class="DigNum (严格)"("Blinking"=w703) -> ()  [unwired: 2 in, 2 out]
            n433 = property on="右180°外全行程间隙" class="DigNum (严格)"("Blinking"=w702) -> ()  [unwired: 2 in, 2 out]
            n434 = Add(x=w721, y=-10.0) -> (x+y=w722:dbl)
          }
          frame #14 {
            n435 = Compound Arithmetic op=OR(w733, w732, w731, w730) -> (w729:bool)
            n436 = property on="右最大轴向力(N)" class="DigNum (严格)"("Blinking"=w736) -> ()  [unwired: 2 in, 2 out]
            n437 = property on="右平均轴向力(N)" class="DigNum (严格)"("Blinking"=w735) -> ()  [unwired: 2 in, 2 out]
            n438 = property on="右轴向力波动(N)" class="DigNum (严格)"("Blinking"=w734) -> ()  [unwired: 2 in, 2 out]
            n439 = Compound Arithmetic op=OR(w727, w729, w736, w735, w734, w739, w738, w737, w728) -> (w741:bool)
            n440 = Not(x=w741) -> (.not. x?=w740:bool)
            n441 = local write "轴向力及全行程间隙合格"(w740) -> ()
          }
          frame #15 {
            n442 = while {
              tunnel: w748 -> [w752]
              tunnel: [w750] -> w747
              tunnel: w746 -> [w749]
              stop <- w751 stop-if-true
              n443 = call "PCI1240电动缸位置模式 .vi"("Distance"=w749, "AxisHandle IN"=w752) -> ("AbsSuccess"=w751:bool, "AxisHandle OUT"=w750:u32)  [unwired: 8 in]
              n444 = Wait (ms)(milliseconds to wait=u32 50 ("毫秒倍数")) -> ()  [unwired: 1 out]
            }
          }
          frame #16 {
            n445 = while {
              tunnel: w755 -> [w759]
              stop <- w757 stop-if-true
              n446 = call <userlib>:"Acm_AxGetCmdVelocity.vi"("AxisHandle"=w759) -> ("Velocity"=w758:dbl)  [unwired: 1 in, 3 out]
              n447 = Wait Until Next ms Multiple(millisecond multiple=u32 50 ("毫秒倍数")) -> ()  [unwired: 1 out]
              n448 = Equal To 0?(x=w758) -> (x = 0?=w757:bool)
            }
          }
          frame #17 {
            n449 = while {
              tunnel: w762 -> [w766]
              tunnel: [w764] -> w761
              tunnel: w760 -> [w763]
              stop <- w765 stop-if-true
              n450 = call "PCI1240电动缸位置模式 .vi"("Distance"=w763, "AxisHandle IN"=w766) -> ("AbsSuccess"=w765:bool, "AxisHandle OUT"=w764:u32)  [unwired: 8 in]
              n451 = Wait (ms)(milliseconds to wait=u32 50 ("毫秒倍数")) -> ()  [unwired: 1 out]
            }
          }
          frame #18 {
            n452 = while {
              tunnel: w768 -> [w772]
              stop <- w770 stop-if-true
              n453 = call <userlib>:"Acm_AxGetCmdVelocity.vi"("AxisHandle"=w772) -> ("Velocity"=w771:dbl)  [unwired: 1 in, 3 out]
              n454 = Wait Until Next ms Multiple(millisecond multiple=u32 50 ("毫秒倍数")) -> ()  [unwired: 1 out]
              n455 = Equal To 0?(x=w771) -> (x = 0?=w770:bool)
            }
          }
          frame #19 {
            n456 = local read "轴向力已做次数"() -> (w775:dbl)
            n457 = Add(x=w775, y=1.0) -> (x+y=w773:dbl)
            n458 = local write "轴向力已做次数"(w773) -> ()
          }
          frame #20 {
            n459 = local read "轴向力及全行程间隙合格"() -> (w776:bool)
            n460 = case shown="假" w776 {
              frame False {
                n461 = Less?(x="轴向力已做次数", y="轴向力设定次数") -> (x < y?=w778:bool)
                n462 = case shown="真" w778 {
                  frame False {
                    n463 = local write "工步号"(u32 45 ("工步号")) -> ()
                  }
                  frame True {
                    n464 = local write "工步号"(u32 30 ("工步号")) -> ()
                  }
                }
              }
              frame True {
                n465 = local write "工步号"(u32 45 ("工步号")) -> ()
              }
            }
          }
        }
      }
      frame 45 {
        # "测头退回"
        n466 = flat-sequence {
          tunnel: [w786] -> w783
          tunnel: w783 -> [w793]
          frame #0 {
            n467 = local write "测头机构轴速度(mm/s)"(30.0 ("测头机构轴速度(mm/s)")) -> ()
          }
          frame #1 {
            n468 = local read "测头机构轴后退位"() -> (w785:dbl)
            n469 = local read "测头机构电机"() -> (w787:u32)
            n470 = while {
              tunnel: w787 -> [w791]
              tunnel: w785 -> [w790]
              tunnel: [w789] -> w786
              stop <- w792 stop-if-true
              n471 = Wait Until Next ms Multiple(millisecond multiple=u32 50 ("毫秒倍数")) -> ()  [unwired: 1 out]
              n472 = call "PCI1220U进给轴位置模式.vi"("Distance"=w790, "AxisHandle IN"=w791) -> ("AbsSuccess"=w792:bool, "AxisHandle OUT"=w789:u32)  [unwired: 8 in]
            }
          }
          frame #2 {
            n473 = while {
              tunnel: w793 -> [w797]
              stop <- w795 stop-if-true
              n474 = call <userlib>:"Acm_AxGetCmdVelocity.vi"("AxisHandle"=w797) -> ("Velocity"=w796:dbl)  [unwired: 1 in, 3 out]
              n475 = Wait Until Next ms Multiple(millisecond multiple=u32 50 ("毫秒倍数")) -> ()  [unwired: 1 out]
              n476 = Equal To 0?(x=w796) -> (x = 0?=w795:bool)
            }
          }
          frame #3 {
            n477 = while {
              stop <- w799 stop-if-true
              n478 = local read "测头机构轴位置(mm)"() -> (w801:dbl)
              n479 = Wait Until Next ms Multiple(millisecond multiple=u32 50 ("毫秒倍数")) -> ()  [unwired: 1 out]
              n480 = Less Or Equal?(x=w801, y=35.0) -> (x <= y?=w799:bool)
            }
          }
          frame #4 {
            n481 = local write "测头气缸右移"(FALSE ("测头气缸右移")) -> ()
            n482 = local write "测头气缸左移"(TRUE ("测头气缸左移")) -> ()
          }
          frame #5 {
            n483 = Wait Until Next ms Multiple(millisecond multiple=u32 500 ("毫秒倍数")) -> ()  [unwired: 1 out]
          }
          frame #6 {
            n484 = local write "工步号"(u32 50 ("工步号")) -> ()
          }
        }
      }
      frame 50 {
        n485 = flat-sequence {
          tunnel: [w828] -> w817
          tunnel: w817 -> [w835]
          tunnel: [w834] -> w814
          tunnel: w814 -> [w846]
          tunnel: [w852] -> w811
          tunnel: w811 -> [w855]
          tunnel: [w854] -> w810
          tunnel: w810 -> [w859]
          tunnel: [w859] -> w809
          tunnel: w809 -> [w861]
          tunnel: [w860] -> w807
          tunnel: [w867] -> w808
          tunnel: w807 -> [w868]
          tunnel: w808 -> [w870]
          tunnel: [w869] -> w806
          tunnel: [w876] -> w816
          tunnel: w806 -> [w876]
          tunnel: w816 -> [w879]
          tunnel: [w878] -> w815
          tunnel: w815 -> [w885]
          tunnel: [w886] -> w813
          tunnel: w813 -> [w893]
          tunnel: [w892] -> w812
          tunnel: w812 -> [w903]
          frame #0 {
            n486 = local write "旋转齿条轴速度(°/s)"(15.0 ("调整螺塞轴速度(°/s)")) -> ()
            n487 = local write "测头机构轴速度(mm/s)"(15.0 ("调整机构轴速度(mm/s)")) -> ()
            n488 = local write "电动缸速度(mm/s)"(15.0 ("电动缸速度(mm/s)")) -> ()
            n489 = local write "夹头夹紧"(FALSE ("夹头夹紧")) -> ()
            n490 = local write "夹头松开"(TRUE ("夹头松开")) -> ()
          }
          frame #1 {
            n491 = while {
              stop <- w823 stop-if-true
              n492 = local read "夹头松开"() -> (w824:bool)
              n493 = local read "夹头夹紧"() -> (w826:bool)
              n494 = Wait Until Next ms Multiple(millisecond multiple=u32 50 ("毫秒倍数")) -> ()  [unwired: 1 out]
              n495 = Not(x=w826) -> (.not. x?=w825:bool)
              n496 = And(x=w825, y=w824) -> (x .and. y?=w823:bool)
            }
          }
          frame #2 {
            n497 = while {
              tunnel: [w831] -> w828
              stop <- w830 stop-if-true
              n498 = local read "电动缸电机"() -> (w832:u32)
              n499 = Wait Until Next ms Multiple(millisecond multiple=u32 50 ("毫秒倍数")) -> ()  [unwired: 1 out]
              n500 = local read "齿条右极限"() -> (w829:dbl)
              n501 = call "PCI1240电动缸位置模式 .vi"("Distance"=w829, "AxisHandle IN"=w832) -> ("AbsSuccess"=w830:bool, "AxisHandle OUT"=w831:u32)  [unwired: 8 in]
            }
          }
          frame #3 {
            n502 = while {
              tunnel: w835 -> [w844]
              tunnel: [w836] -> w834
              stop <- w837 stop-if-true
              n503 = local read "齿条推拉力(N)"() -> (w842:dbl)
              n504 = Wait Until Next ms Multiple(millisecond multiple=u32 50 ("毫秒倍数")) -> ()  [unwired: 1 out]
              n505 = call <userlib>:"Acm_AxGetCmdVelocity.vi"("AxisHandle"=w844) -> ("Velocity"=w845:dbl, "AxisHandle"=w836:u32)  [unwired: 1 in, 2 out]
              n506 = Equal To 0?(x=w845) -> (x = 0?=w839:bool)
              n507 = Absolute Value(x=w842) -> (abs(x)=w841:dbl)
              n508 = Greater Or Equal?(x=w841, y=1000.0) -> (x >= y?=w838:bool)
              n509 = Or(x=w839, y=w838) -> (x .or. y?=w837:bool)
            }
          }
          frame #4 {
            n510 = while {
              tunnel: w846 -> [w850]
              tunnel: [w849] -> _
              stop <- w848 stop-if-true
              n511 = call "PCI1220U停止.vi"("AxisHandle IN"=w850) -> ("完成"=w848:bool, "AxisHandle OUT"=w849:u32)  [unwired: 9 in]
              n512 = Wait (ms)(milliseconds to wait=u32 50 ("毫秒倍数")) -> ()  [unwired: 1 out]
            }
          }
          frame #5 {
            n513 = local write "旋转齿条轴使能"(TRUE ("旋转齿条轴使能")) -> ()
          }
          frame #6 {
            n514 = local read "旋转齿条电机"() -> (w852:u32)
            n515 = Wait Until Next ms Multiple(millisecond multiple=u32 500 ("毫秒倍数")) -> ()  [unwired: 1 out]
          }
          frame #7 {
            n516 = call <userlib>:"Acm_AxHome.vi"("DirMode"=u32 0, "HomeMode"=u32 11, "AxisHandle"=w855) -> ("AxisHandle"=w854:u32)  [unwired: 1 in, 2 out]
          }
          frame #8 {
            n517 = Wait Until Next ms Multiple(millisecond multiple=u32 100 ("毫秒倍数")) -> ()  [unwired: 1 out]
          }
          frame #9 {
            n518 = while {
              tunnel: w861 -> [w864]
              tunnel: [w863] -> w860
              stop <- w862 stop-if-true
              n519 = call <userlib>:"Acm_AxGetCmdVelocity.vi"("AxisHandle"=w864) -> ("Velocity"=w866:dbl, "AxisHandle"=w863:u32)  [unwired: 1 in, 2 out]
              n520 = Wait Until Next ms Multiple(millisecond multiple=u32 50 ("毫秒倍数")) -> ()  [unwired: 1 out]
              n521 = Equal To 0?(x=w866) -> (x = 0?=w862:bool)
            }
          }
          frame #10 {
            n522 = call "PCI1220U角度置零.vi"("AxisHandle IN"=w868) -> ("AxisHandle OUT"=w867:u32)  [unwired: 10 in]
          }
          frame #11 {
            n523 = while {
              tunnel: w870 -> [w872]
              tunnel: [w871] -> w869
              stop <- w875 stop-if-true
              n524 = Wait Until Next ms Multiple(millisecond multiple=u32 50 ("毫秒倍数")) -> ()  [unwired: 1 out]
              n525 = call "PCI1220U扭矩轴位置模式.vi"("Distance"=10.0, "AxisHandle IN"=w872) -> ("AbsSuccess"=w875:bool, "AxisHandle OUT"=w871:u32)  [unwired: 8 in]
            }
          }
          frame #12 {
            n526 = Wait Until Next ms Multiple(millisecond multiple=u32 500 ("毫秒倍数")) -> ()  [unwired: 1 out]
          }
          frame #13 {
            n527 = while {
              tunnel: w879 -> [w882]
              tunnel: [w881] -> w878
              stop <- w880 stop-if-true
              n528 = call <userlib>:"Acm_AxGetCmdVelocity.vi"("AxisHandle"=w882) -> ("Velocity"=w884:dbl, "AxisHandle"=w881:u32)  [unwired: 1 in, 2 out]
              n529 = Wait Until Next ms Multiple(millisecond multiple=u32 50 ("毫秒倍数")) -> ()  [unwired: 1 out]
              n530 = Equal To 0?(x=w884) -> (x = 0?=w880:bool)
            }
          }
          frame #14 {
            n531 = call "PCI1220U角度置零.vi"("AxisHandle IN"=w885) -> ()  [unwired: 10 in, 1 out]
          }
          frame #15 {
            n532 = while {
              tunnel: [w889] -> w886
              stop <- w888 stop-if-true
              n533 = local read "电动缸电机"() -> (w890:u32)
              n534 = Wait Until Next ms Multiple(millisecond multiple=u32 50 ("毫秒倍数")) -> ()  [unwired: 1 out]
              n535 = local read "齿条右极限"() -> (w887:dbl)
              n536 = call "PCI1240电动缸位置模式 .vi"("Distance"=w887, "AxisHandle IN"=w890) -> ("AbsSuccess"=w888:bool, "AxisHandle OUT"=w889:u32)  [unwired: 8 in]
            }
          }
          frame #16 {
            n537 = while {
              tunnel: w893 -> [w901]
              tunnel: [w899] -> w892
              stop <- w894 stop-if-true
              n538 = local read "齿条推拉力(N)"() -> (w898:dbl)
              n539 = Wait Until Next ms Multiple(millisecond multiple=u32 50 ("毫秒倍数")) -> ()  [unwired: 1 out]
              n540 = call <userlib>:"Acm_AxGetCmdVelocity.vi"("AxisHandle"=w901) -> ("Velocity"=w902:dbl, "AxisHandle"=w899:u32)  [unwired: 1 in, 2 out]
              n541 = Equal To 0?(x=w902) -> (x = 0?=w896:bool)
              n542 = Greater Or Equal?(x=w898, y=300.0) -> (x >= y?=w895:bool)
              n543 = Or(x=w896, y=w895) -> (x .or. y?=w894:bool)
            }
          }
          frame #17 {
            n544 = while {
              tunnel: w903 -> [w907]
              tunnel: [w906] -> _
              stop <- w905 stop-if-true
              n545 = call "PCI1220U停止.vi"("AxisHandle IN"=w907) -> ("完成"=w905:bool, "AxisHandle OUT"=w906:u32)  [unwired: 9 in]
              n546 = Wait (ms)(milliseconds to wait=u32 50 ("毫秒倍数")) -> ()  [unwired: 1 out]
            }
          }
          frame #18 {
            n547 = local write "工步号"(u32 100 ("工步号")) -> ()
          }
        }
      }
      frame 100 {
        n548 = flat-sequence {
          tunnel: [w942] -> w932
          tunnel: [w940] -> w931
          tunnel: [w934] -> w919
          tunnel: [w933] -> w916
          tunnel: w932 -> [w949]
          tunnel: w931 -> [w946]
          tunnel: ["F:\\报表存储\\" ("字符串")] -> w930
          tunnel: w919 -> [w948]
          tunnel: [w949] -> w918
          tunnel: [w948] -> w917
          tunnel: w916 -> [w947]
          tunnel: [w947] -> w915
          tunnel: [w946] -> w914
          tunnel: w930 -> [w961]
          tunnel: [w968] -> w929
          tunnel: [w966] -> w928
          tunnel: [w965] -> w927
          tunnel: [w964] -> w926
          tunnel: w918 -> [w960]
          tunnel: w917 -> [w959]
          tunnel: w915 -> [w958]
          tunnel: w914 -> [w951]
          tunnel: [w953] -> w909
          tunnel: w929 -> [w975]
          tunnel: [w976] -> w925
          tunnel: w928 -> [w976]
          tunnel: w927 -> [w974]
          tunnel: w926 -> [w973]
          tunnel: [w972] -> w924
          tunnel: [w971] -> w923
          tunnel: [w970] -> w910
          tunnel: w909 -> [w970]
          tunnel: [w983] -> w922
          tunnel: w925 -> [w983]
          tunnel: w924 -> [w982]
          tunnel: [w982] -> w921
          tunnel: [w981] -> w920
          tunnel: w923 -> [w981]
          tunnel: [w979] -> w911
          tunnel: w910 -> [w979]
          tunnel: w922 -> [w986]
          tunnel: w921 -> [w994]
          tunnel: w920 -> [w993]
          tunnel: [w985] -> w912
          tunnel: w911 -> [w985]
          tunnel: [w1002] -> w913
          tunnel: w912 -> [w1002]
          tunnel: w913 -> [w1004]
          frame #0 {
            n549 = local read "产品ID"() -> (w941:string)
            n550 = Format Date/Time String(time format string (%c)="%Y%m%d" ("时间格式字符串(%c)")) -> (date/time string=w935:string)  [unwired: 2 in]
            n551 = String Subset(string=w935, offset (0)=6 ("偏移量(0)"), length (rest)=2 ("长度（剩余）")) -> (substring=w933:string)
            n552 = String Subset(string=w935, offset (0)=4 ("偏移量(0)"), length (rest)=2 ("长度（剩余）")) -> (substring=w934:string)
            n553 = String Subset(string=w935, offset (0)=0 ("偏移量(0)"), length (rest)=4 ("长度（剩余）")) -> (substring=w942:string)
            n554 = call <vilib>:"Trim Whitespace.vi"("string"=w941) -> ("trimmed string"=w940:string)  [unwired: 1 in]
          }
          frame #1 {
          }
          frame #2 {
            w952 = "\\" ("字符串")
            n555 = Concatenate Strings(w961, w960, w952, w959, w952, w958, w952, w951, w952) -> (w955:string)
            n556 = Concatenate Strings(w961, w960, w952, w959, w952, w958, w952, w951, w952) -> (w969:string)
            n557 = Concatenate Strings(w955, w951, "间隙曲线.JPG" ("字符串")) -> (w967:string)
            n558 = Concatenate Strings(w955, "轴向力曲线数组.txt" ("字符串")) -> (w964:string)
            n559 = Concatenate Strings(w955, "扭动曲线数组.txt" ("字符串")) -> (w965:string)
            n560 = Concatenate Strings(w955, w951, "轴向力曲线.JPG" ("字符串")) -> (w957:string)
            n561 = String To Path(string=w967) -> (path=w966:path)
            n562 = String To Path(string=w969) -> (path=w968:path)
            n563 = String To Path(string=w957) -> (path=w953:path)
          }
          frame #3 {
            n564 = call <vilib>:"Check if File or Folder Exists.vi"("path"=w975) -> ("file or folder exists?"=w977:bool)  [unwired: 8 in, 2 out]
            n565 = case shown="假" w977 {
              tunnel: w975 -> [w978 _]
              frame False {
                n566 = Create Folder(path (use dialog)=w978) -> ()  [unwired: 2 in, 3 out]
              }
              frame True {
              }
            }
            n567 = String To Path(string=w973) -> (path=w971:path)
            n568 = String To Path(string=w974) -> (path=w972:path)
          }
          frame #4 {
            n569 = local write "选项卡控件"(T1."间隙测量" ("选项卡控件")) -> ()
            n570 = Wait Until Next ms Multiple(millisecond multiple=u32 1000 ("毫秒倍数")) -> ()  [unwired: 1 out]
          }
          frame #5 {
            n571 = disable-structure shown="禁用" {
              disable-tunnel: w986 -> [w995 _]
              frame Disabled {
                w999 = T2 2 items=["快速打印", "标准报表", "HTML", "双字节", "Excel"] ("report type (Quick Print)")
                w998 = T3 1 items=["完整前面板", "前面板可见部分", "图标、说明、前面板和程序框图", "说明信息: 使用前面板", "说明信息: 作为子VI使用", "说明信息: 完整", "说明信息: 自定义"] ("contents (complete front panel)")
                n572 = Current VI's Path() -> (path=w997:path)
                n573 = call-poly <vilib>:"Easy Print VI Panel or Documentation.vi"("report type (Quick Print)"=w999, "contents (complete front panel)"=w998, "VI path"=w997) -> ("error out"=w1001:errorcluster, "report out"=w1000:refnum<class "NI_report.lvclass">)  [unwired: 1 in, 6 out]
                n574 = call-dynamic "Save Report to File.vi"("report in"=w1000, "report file path"=w995, "error in (no error)"=w1001) -> ("error out"=→"error out 3":errorcluster)  [unwired: 2 in, 10 out]
              }
              frame Enabled {
              }
            }
            n575 = local read "间隙Y数组"() -> (w991:dbl[])
            n576 = local read "间隙X数组"() -> (w992:dbl[])
            n577 = local read "轴向力Y"() -> (w989:dbl[])
            n578 = local read "轴向力X"() -> (w990:dbl[])
            n579 = call "导出曲线数组.vi"("file path (dialog if empty)"=w994, "数组 2"=w991, "数组"=w992) -> ()  [unwired: 9 in]
            n580 = call "导出曲线数组.vi"("file path (dialog if empty)"=w993, "数组 2"=w989, "数组"=w990) -> ()  [unwired: 9 in]
            n581 = control-ref of="本VI"() -> (w988:refnum<vi>)
            n582 = invoke class="VI" method="FP.Get Image"(reference=w988) -> ("image data"=w987:T4)  [unwired: 5 in, 5 out]
            n583 = call <vilib>:"Write JPEG File.vi"("image data"=w987, "path to JPEG file"=w986) -> ()  [unwired: 8 in, 2 out]
          }
          frame #6 {
            n584 = local write "选项卡控件"(T1."轴向力测量" ("选项卡控件")) -> ()
          }
          frame #7 {
            n585 = control-ref of="本VI"() -> (w1005:refnum<vi>)
            n586 = invoke class="VI" method="FP.Get Image"(reference=w1005) -> ("image data"=w1006:T4)  [unwired: 5 in, 5 out]
            n587 = call <vilib>:"Write JPEG File.vi"("image data"=w1006, "path to JPEG file"=w1004) -> ()  [unwired: 8 in, 2 out]
          }
          frame #8 {
            n588 = local read "联线按钮"() -> (w1007:bool)
            n589 = case shown="真" w1007 {
              frame False {
              }
              frame True {
                n590 = flat-sequence {
                  tunnel: [w1010] -> w1008
                  tunnel: [w1018] -> w1009
                  tunnel: w1008 -> [w1014]
                  tunnel: w1009 -> [w1032]
                  frame #0 {
                    n591 = local read "轴向力及全行程间隙合格"() -> (w1011:bool)
                    n592 = local read "单点间隙合格"() -> (w1012:bool)
                    n593 = And(x=w1012, y=w1011) -> (x .and. y?=w1010:bool)
                  }
                  frame #1 {
                    n594 = local read "左全行程间隙"() -> (w1021:dbl)
                    n595 = Boolean To (0,1)(Boolean=w1014) -> (0, 1=w1016:i16)
                    n596 = local read "中间位置间隙"() -> (w1024:dbl)
                    n597 = local read "员工ID"() -> (w1029:string)
                    n598 = local read "FGCS"() -> (w1026:string)
                    n599 = local read "KSJJ"() -> (w1028:string)
                    n600 = local read "产品ID"() -> (w1030:string)
                    n601 = Number To Decimal String(number=w1016, width (-)=i16 1 ("宽度(-)")) -> (decimal integer string=w1013:string)
                    n602 = Format Date/Time String(time format string (%c)="%Y%m%d%H%M" ("时间格式字符串(%c)")) -> (date/time string=w1027:string)  [unwired: 2 in]
                    n603 = Number To Fractional String(number=w1021, precision (6)=i16 3 ("精度(6)")) -> (F-format string=w1019:string)  [unwired: 2 in]
                    n604 = Number To Fractional String(number=w1024, precision (6)=i16 3 ("精度(6)")) -> (F-format string=w1020:string)  [unwired: 2 in]
                    n605 = Build Array(w1030, w1029, "1", w1013, w1028, w1027, w1026, "Q14073-11A", w1020, w1019) -> (w1018:string[])
                  }
                  frame #2 {
                    n606 = Wait (ms)(milliseconds to wait=u32 500 ("等待时间（毫秒）")) -> ()  [unwired: 1 out]
                    n607 = call "数据库更新.vi"("设备号"="06", "数据"=w1032) -> ()  [unwired: 13 in, 1 out]
                  }
                  frame #3 {
                  }
                }
              }
            }
          }
          frame #9 {
            n608 = local write "产品ID"("") -> ()
            n609 = local write "工步号"(u32 0 ("工步号")) -> ()
          }
        }
      }
    }
    n610 = Wait (ms)(milliseconds to wait=u32 50 ("毫秒倍数")) -> ()  [unwired: 1 out]
    n611 = local read "停止"() -> (w7:bool)
  }
  n612 = while {
    stop <- w1037 stop-if-true
    n613 = event shown="[2] \"参数修改\": 值改变" {
      selector: _ -> [_ _ _ _ _ _ _]
      dyn-events: _ -> [_ _ _ _ _ _ _]
      timeout: 500 -> [_ _ _ _ _ _ _]
      event Timeout {
        n614 = event-data() -> ()  [unwired: 3 out]
      }
      event "停止": Value Change {
        n615 = event-data() -> ()  [unwired: 6 out]
        n616 = flat-sequence {
          frame #0 {
            n617 = Wait (ms)(milliseconds to wait=u32 1000 ("毫秒倍数")) -> ()  [unwired: 1 out]
          }
          frame #1 {
            n618 = Quit LabVIEW(quit? (T)=TRUE ("停止？(T)")) -> ()
          }
        }
      }
      event "参数修改": Value Change {
        n619 = event-data() -> ()  [unwired: 6 out]
        n620 = while {
          i -> [w1044]
          stop <- w1043 stop-if-true
          n621 = local read "型号数量"() -> (w1045:i32)
          n622 = local read "参数浏览表"() -> (w1046:string[][])
          n623 = Wait Until Next ms Multiple(millisecond multiple=u32 50 ("毫秒倍数")) -> ()  [unwired: 1 out]
          n624 = Greater Or Equal?(x=w1044, y=w1045) -> (x >= y?=w1043:bool)
          n625 = Index Array(array=w1046, index (col)=w1044) -> (element=w1042:string[])  [unwired: 1 in]
          n626 = stacked-sequence {
            tunnel: w1042 -> [w1080]
            frame #0 {
              n627 = Index Array(array=w1080, index #1=0 ("索引"), index #2=2 ("索引"), index #3=3 ("索引"), index #4=4 ("索引"), index #5=5 ("索引"), index #6=6 ("索引"), index #7=7 ("索引"), index #8=8 ("索引"), index #9=9 ("索引"), index #10=10 ("索引"), index #11=11 ("索引"), index #12=12 ("索引"), index #13=13 ("索引"), index #14=14 ("索引"), index #15=15 ("索引"), index #16=16 ("索引"), index #17=17 ("索引"), index #18=18 ("索引"), index #19=19 ("索引")) -> (element #1=w1052:string, element #2=w1076:string, element #3=w1075:string, element #4=w1074:string, element #5=w1073:string, element #6=w1072:string, element #7=w1071:string, element #8=w1070:string, element #9=w1069:string, element #10=w1068:string, element #11=w1067:string, element #12=w1058:string, element #13=w1057:string, element #14=w1056:string, element #15=w1055:string, element #16=w1054:string, element #17=w1053:string, element #18=w1049:string, element #19=w1048:string)
              n628 = call "创建文本"("测头机构轴移动速度"=w1076, "测头机构轴检测位"=w1075, "测头机构轴待检位"=w1074, "测头机构轴后退位"=w1073, "齿条移动速度"=w1072, "齿条左极限"=w1071, "齿条右极限"=w1070, "旋转齿条轴找帽转速"=w1069, "旋转齿条轴测量转速"=w1068, "测量点扭矩"=w1067, "总行程最小值"=w1058, "总行程最大值"=w1057, "最大轴向力"=w1056, "轴向力波动"=w1055, "平均轴向力最小值"=w1054, "平均轴向力最大值"=w1053, "总圈数最小值"=w1049, "总圈数最大值"=w1048, "产品型号"=w1052) -> ("Result"=w1066:string)  [unwired: 7 in, 1 out]
              n629 = local read "ADODB._Connection Out 2"() -> (w1065:refnum<k7>)
              n630 = call "SQL Execute.vi"("Command Text"=w1066, "ADODB._Connection In"=w1065) -> ("error out"=w1078:errorcluster, "ADODB._Connection Out"=w1079:refnum<k7>)  [unwired: 6 in, 2 out]
              n631 = call "ADO Connection Close.vi"("error in (no error)"=w1078, "ADODB._Connection In"=w1079) -> ("error out"=→"error out":errorcluster)  [unwired: 8 in, 1 out]
            }
          }
        }
      }
      event "参数查询": Value Change {
        n632 = event-data() -> ()  [unwired: 6 out]
        n633 = flat-sequence {
          tunnel: [w1103] -> w1096
          tunnel: [w1102] -> w1095
          tunnel: [w1101] -> w1092
          tunnel: w1096 -> [w1107]
          tunnel: w1095 -> [w1109]
          tunnel: [w1109] -> w1094
          tunnel: [w1108] -> w1093
          tunnel: w1092 -> [w1108]
          tunnel: w1094 -> [_]
          tunnel: w1093 -> [_]
          frame #0 {
            n634 = call-poly <vilib>:"Read From Spreadsheet File.vi"("file path (dialog if empty)"=path "D:/Q14070-Z060人机界面/参数/参数项.txt") -> ("first row"=w1097:string[])  [unwired: 6 in, 4 out]
            n635 = property on="参数浏览表" class="Tbl (严格)"("Row Headers[]"=w1097) -> ()  [unwired: 2 in, 2 out]
          }
          frame #1 {
            n636 = local read "ADODB._Connection Out 2"() -> (w1100:refnum<k7>)
            n637 = call "SQL Execute.vi"("Command Text"="SELECT * FROM 测试参数表;", "ADODB._Connection In"=w1100) -> ("error out"=w1101:errorcluster, "Data"=w1105:string[][], "ADODB._Connection Out"=w1102:refnum<k7>)  [unwired: 6 in, 1 out]
            n638 = Transpose 2D Array(2D array=w1105) -> (transposed array=w1103:string[][])
            n639 = Index Array(array=w1103, index (row)=0 ("索引 (行)")) -> (element=w1104:string[])  [unwired: 1 in]
            n640 = property on="参数浏览表" class="Tbl (严格)"("Column Headers[]"=w1104) -> ()  [unwired: 2 in, 2 out]
          }
          frame #2 {
            n641 = local write "参数浏览表"(w1107) -> ()
          }
          frame #3 {
          }
        }
      }
      event "传感器参数保存": Value Change {
        n642 = event-data() -> ()  [unwired: 6 out]
        n643 = flat-sequence {
          tunnel: [w1135] -> w1132
          tunnel: [w1134] -> w1131
          tunnel: [w1133] -> w1130
          tunnel: [w1141] -> w1129
          tunnel: w1132 -> [w1141]
          tunnel: [w1140] -> w1128
          tunnel: w1131 -> [w1140]
          tunnel: [w1139] -> w1127
          tunnel: w1130 -> [w1139]
          tunnel: [w1138] -> w1126
          tunnel: [w1137] -> w1125
          tunnel: [w1136] -> w1124
          tunnel: [w1142] -> w1123
          tunnel: [w1148] -> w1122
          tunnel: w1129 -> [w1148]
          tunnel: [w1147] -> w1121
          tunnel: w1128 -> [w1147]
          tunnel: w1127 -> [w1146]
          tunnel: [w1146] -> w1120
          tunnel: [w1145] -> w1119
          tunnel: w1126 -> [w1145]
          tunnel: [w1144] -> w1118
          tunnel: w1125 -> [w1144]
          tunnel: [w1143] -> w1117
          tunnel: w1124 -> [w1143]
          tunnel: w1123 -> [w1167]
          tunnel: [w1167] -> w1116
          tunnel: w1122 -> [w1166]
          tunnel: w1121 -> [w1159]
          tunnel: w1120 -> [w1158]
          tunnel: w1119 -> [w1152]
          tunnel: w1118 -> [w1151]
          tunnel: w1117 -> [w1157]
          tunnel: [w1156] -> w1115
          tunnel: [w1155] -> w1114
          tunnel: [w1154] -> w1113
          tunnel: [w1150] -> w1112
          tunnel: [w1149] -> w1111
          tunnel: [w1153] -> w1110
          tunnel: w1116 -> [w1175]
          tunnel: w1115 -> [w1174]
          tunnel: w1114 -> [w1173]
          tunnel: w1113 -> [w1172]
          tunnel: w1112 -> [w1171]
          tunnel: w1111 -> [w1170]
          tunnel: w1110 -> [w1169]
          frame #0 {
            n644 = local read "齿条推拉力零点偏移"() -> (w1134:dbl)
            n645 = local read "间隙位移零点偏移"() -> (w1135:dbl)
            n646 = local read "齿条扭矩零点偏移"() -> (w1133:dbl)
          }
          frame #1 {
            n647 = local read "齿条推拉力比例偏移"() -> (w1137:dbl)
            n648 = local read "间隙位移比例偏移"() -> (w1138:dbl)
            n649 = local read "齿条扭矩比例偏移"() -> (w1136:dbl)
          }
          frame #2 {
            n650 = local read "ADODB._Connection Out 2"() -> (w1142:refnum<k7>)
          }
          frame #3 {
            n651 = Number To Fractional String(number=w1166, precision (6)=i16 2 ("精度(6)")) -> (F-format string=w1156:string)  [unwired: 2 in]
            n652 = Number To Fractional String(number=w1158, precision (6)=i16 2 ("精度(6)")) -> (F-format string=w1154:string)  [unwired: 2 in]
            n653 = Number To Fractional String(number=w1157, precision (6)=i16 2 ("精度(6)")) -> (F-format string=w1153:string)  [unwired: 2 in]
            n654 = Number To Fractional String(number=w1159, precision (6)=i16 2 ("精度(6)")) -> (F-format string=w1155:string)  [unwired: 2 in]
            n655 = Number To Fractional String(number=w1152, precision (6)=i16 2 ("精度(6)")) -> (F-format string=w1150:string)  [unwired: 2 in]
            n656 = Number To Fractional String(number=w1151, precision (6)=i16 2 ("精度(6)")) -> (F-format string=w1149:string)  [unwired: 2 in]
          }
          frame #4 {
            n657 = call "创建文本3"("4"=w1171, "6"=w1169, "1"=w1174, "2"=w1173, "3"=w1172, "5"=w1170) -> ("Result"=w1176:string)  [unwired: 8 in, 1 out]
            n658 = call "SQL Execute.vi"("Command Text"=w1176, "ADODB._Connection In"=w1175) -> ("error out"=→"error out 4":errorcluster)  [unwired: 6 in, 3 out]
          }
        }
      }
      event "产品ID": Value Change {
        n659 = event-data() -> ()  [unwired: 7 out]
        n660 = Format Date/Time String(time format string (%c)="%Y%m%d%H%M" ("时间格式字符串(%c)")) -> (date/time string=w1177:string)  [unwired: 2 in]
        n661 = local write "KSJJ"(w1177) -> ()
      }
      event "电动缸回零": Mouse Down {
        n662 = event-data() -> ()  [unwired: 6 out]
        n663 = stacked-sequence {
          frame #0 {
            n664 = flat-sequence {
              tunnel: [w1195] -> w1184
              tunnel: [w1188] -> w1181
              tunnel: w1184 -> [w1198]
              tunnel: [w1198] -> w1183
              tunnel: [w1196] -> w1182
              tunnel: w1181 -> [w1196]
              tunnel: w1183 -> [w1200]
              tunnel: [w1200] -> w1185
              tunnel: w1182 -> [w1199]
              tunnel: [w1199] -> w1180
              tunnel: w1185 -> [w1210]
              tunnel: w1180 -> [w1209]
              frame #0 {
                n665 = local write "电动缸速度(mm/s)"(15.0 ("电动缸速度(mm/s)")) -> ()
                n666 = local write "测头机构轴速度(mm/s)"(10.0 ("电动缸速度(mm/s)")) -> ()
              }
              frame #1 {
                n667 = local read "测头机构电机"() -> (w1192:u32)
                n668 = local read "电动缸电机"() -> (w1189:u32)
                n669 = call <userlib>:"Acm_AxHome.vi"("DirMode"=u32 0, "HomeMode"=u32 11, "AxisHandle"=w1192) -> ("AxisHandle"=w1195:u32)  [unwired: 1 in, 2 out]
                n670 = call <userlib>:"Acm_AxHome.vi"("DirMode"=u32 1, "HomeMode"=u32 11, "AxisHandle"=w1189) -> ("AxisHandle"=w1188:u32)  [unwired: 1 in, 2 out]
              }
              frame #2 {
                n671 = Wait Until Next ms Multiple(millisecond multiple=u32 100 ("毫秒倍数")) -> ()  [unwired: 1 out]
              }
              frame #3 {
                n672 = while {
                  tunnel: w1200 -> [w1208]
                  stop <- w1206 stop-if-true
                  n673 = call <userlib>:"Acm_AxGetCmdVelocity.vi"("AxisHandle"=w1208) -> ("Velocity"=w1207:dbl)  [unwired: 1 in, 3 out]
                  n674 = Wait Until Next ms Multiple(millisecond multiple=u32 50 ("毫秒倍数")) -> ()  [unwired: 1 out]
                  n675 = Equal To 0?(x=w1207) -> (x = 0?=w1206:bool)
                }
                n676 = while {
                  tunnel: w1199 -> [w1204]
                  stop <- w1202 stop-if-true
                  n677 = call <userlib>:"Acm_AxGetCmdVelocity.vi"("AxisHandle"=w1204) -> ("Velocity"=w1203:dbl)  [unwired: 1 in, 3 out]
                  n678 = Wait Until Next ms Multiple(millisecond multiple=u32 50 ("毫秒倍数")) -> ()  [unwired: 1 out]
                  n679 = Equal To 0?(x=w1203) -> (x = 0?=w1202:bool)
                }
              }
              frame #4 {
                n680 = call "PCI1220U角度置零.vi"("AxisHandle IN"=w1210) -> ()  [unwired: 10 in, 1 out]
                n681 = call "PCI1220U角度置零.vi"("AxisHandle IN"=w1209) -> ()  [unwired: 10 in, 1 out]
              }
              frame #5 {
              }
              frame #6 {
              }
            }
          }
          frame #1 {
            n682 = flat-sequence {
              tunnel: [w1222] -> w1217
              tunnel: w1217 -> [w1224]
              tunnel: [w1224] -> w1216
              tunnel: w1216 -> [w1225]
              tunnel: [w1225] -> w1215
              tunnel: w1215 -> [w1231]
              tunnel: [w1230] -> w1212
              tunnel: w1212 -> [w1233]
              tunnel: [w1233] -> w1211
              tunnel: w1211 -> [w1235]
              tunnel: [w1234] -> w1214
              tunnel: w1214 -> [w1241]
              tunnel: [w1241] -> w1213
              tunnel: w1213 -> [w1246]
              frame #0 {
                n683 = local write "旋转齿条轴速度(°/s)"(5.0 ("电动缸速度(mm/s)")) -> ()
              }
              frame #1 {
                n684 = local read "旋转齿条电机"() -> (w1219:u32)
                n685 = call <userlib>:"Acm_AxHome.vi"("DirMode"=u32 0, "HomeMode"=u32 11, "AxisHandle"=w1219) -> ("AxisHandle"=w1222:u32)  [unwired: 1 in, 2 out]
              }
              frame #2 {
                n686 = Wait Until Next ms Multiple(millisecond multiple=u32 100 ("毫秒倍数")) -> ()  [unwired: 1 out]
              }
              frame #3 {
                n687 = while {
                  tunnel: w1225 -> [w1229]
                  stop <- w1227 stop-if-true
                  n688 = call <userlib>:"Acm_AxGetCmdVelocity.vi"("AxisHandle"=w1229) -> ("Velocity"=w1228:dbl)  [unwired: 1 in, 3 out]
                  n689 = Wait Until Next ms Multiple(millisecond multiple=u32 50 ("毫秒倍数")) -> ()  [unwired: 1 out]
                  n690 = Equal To 0?(x=w1228) -> (x = 0?=w1227:bool)
                }
              }
              frame #4 {
                n691 = call "PCI1220U角度置零.vi"("AxisHandle IN"=w1231) -> ("AxisHandle OUT"=w1230:u32)  [unwired: 10 in]
              }
              frame #5 {
                n692 = Wait (ms)(milliseconds to wait=u32 100 ("等待时间（毫秒）")) -> ()  [unwired: 1 out]
              }
              frame #6 {
                n693 = while {
                  tunnel: [w1239] -> w1234
                  tunnel: w1235 -> [w1236]
                  stop <- w1238 stop-if-true
                  n694 = Wait Until Next ms Multiple(millisecond multiple=u32 50 ("毫秒倍数")) -> ()  [unwired: 1 out]
                  n695 = call "PCI1220U扭矩轴位置模式.vi"("Distance"=10.0, "AxisHandle IN"=w1236) -> ("AbsSuccess"=w1238:bool, "AxisHandle OUT"=w1239:u32)  [unwired: 8 in]
                }
              }
              frame #7 {
                n696 = while {
                  tunnel: w1241 -> [w1244]
                  stop <- w1242 stop-if-true
                  n697 = call <userlib>:"Acm_AxGetCmdVelocity.vi"("AxisHandle"=w1244) -> ("Velocity"=w1245:dbl)  [unwired: 1 in, 3 out]
                  n698 = Wait Until Next ms Multiple(millisecond multiple=u32 50 ("毫秒倍数")) -> ()  [unwired: 1 out]
                  n699 = Equal To 0?(x=w1245) -> (x = 0?=w1242:bool)
                }
              }
              frame #8 {
                n700 = call "PCI1220U角度置零.vi"("AxisHandle IN"=w1246) -> ()  [unwired: 10 in, 1 out]
              }
            }
          }
          frame #2 {
            n701 = flat-sequence {
              frame #0 {
                n702 = while {
                  stop <- w1250 stop-if-true
                  n703 = local read "电动缸回零"() -> (w1251:bool)
                  n704 = local write "回零完成"(TRUE ("回零完成")) -> ()
                  n705 = local write "电动缸回零"(FALSE ("电动缸回零")) -> ()
                  n706 = Wait Until Next ms Multiple(millisecond multiple=u32 50 ("毫秒倍数")) -> ()  [unwired: 1 out]
                  n707 = Not(x=w1251) -> (.not. x?=w1250:bool)
                }
              }
            }
          }
        }
        n708 = Wait Until Next ms Multiple(millisecond multiple=u32 50 ("毫秒倍数")) -> ()  [unwired: 1 out]
      }
    }
    n709 = Wait (ms)(milliseconds to wait=u32 50 ("毫秒倍数")) -> ()  [unwired: 1 out]
    n710 = local read "停止"() -> (w1037:bool)
  }
  n711 = call "PCI1240电动缸位置模式 .vi"() -> ()  [unwired: 10 in, 2 out]
  n712 = while {
    stop <- w1253 stop-if-true
    n713 = stacked-sequence {
      frame #0 {
        n714 = flat-sequence {
          frame #0 {
          }
          frame #1 {
          }
          frame #2 {
            n715 = First Call?() -> (First Call?: T/F=w1254:bool)
            n716 = case shown="真" w1254 {
              frame False {
              }
              frame True {
                n717 = call "员工管理测试程序.vi"() -> ("员工姓名"=w1256:string, "员工ID"=w1255:string)  [unwired: 10 in]
                n718 = local write "员工ID"(w1255) -> ()
                n719 = local write "员工姓名"(w1256) -> ()
              }
            }
          }
          frame #3 {
          }
          frame #4 {
          }
          frame #5 {
          }
          frame #6 {
          }
        }
      }
      frame #1 {
        n720 = flat-sequence {
          frame #0 {
            n721 = property on="型号选择" class="Ring (严格)"() -> ("RingText.Text"=w1257:string)  [unwired: 2 in, 2 out]
            n722 = case shown="\"J706\"" w1257 {
              frame "J709", Default {
                w1258 = FALSE ("可见")
                w1259 = TRUE ("可见")
                n723 = property on="右180°内全行程间隙" class="DigNum (严格)"("Visible"=w1258) -> ()  [unwired: 2 in, 2 out]
                n724 = property on="右180°外全行程间隙" class="DigNum (严格)"("Visible"=w1258) -> ()  [unwired: 2 in, 2 out]
                n725 = property on="左180°外全行程间隙" class="DigNum (严格)"("Visible"=w1258) -> ()  [unwired: 2 in, 2 out]
                n726 = property on="左180°内全行程间隙" class="DigNum (严格)"("Visible"=w1258) -> ()  [unwired: 2 in, 2 out]
                n727 = property on="右全行程间隙" class="DigNum (严格)"("Visible"=w1259) -> ()  [unwired: 2 in, 2 out]
                n728 = property on="左全行程间隙" class="DigNum (严格)"("Visible"=w1259) -> ()  [unwired: 2 in, 2 out]
              }
              frame "J706" {
                w1260 = TRUE ("可见")
                w1261 = FALSE ("可见")
                n729 = property on="右180°内全行程间隙" class="DigNum (严格)"("Visible"=w1260) -> ()  [unwired: 2 in, 2 out]
                n730 = property on="右180°外全行程间隙" class="DigNum (严格)"("Visible"=w1260) -> ()  [unwired: 2 in, 2 out]
                n731 = property on="左180°外全行程间隙" class="DigNum (严格)"("Visible"=w1260) -> ()  [unwired: 2 in, 2 out]
                n732 = property on="左180°内全行程间隙" class="DigNum (严格)"("Visible"=w1260) -> ()  [unwired: 2 in, 2 out]
                n733 = property on="右全行程间隙" class="DigNum (严格)"("Visible"=w1261) -> ()  [unwired: 2 in, 2 out]
                n734 = property on="左全行程间隙" class="DigNum (严格)"("Visible"=w1261) -> ()  [unwired: 2 in, 2 out]
              }
            }
          }
          frame #1 {
            (unwired) string[] ["I急停按钮", "I自动旋钮", "I启动按钮", "I备用按钮", "I复位按钮", "I上阻挡器放行", "I下阻挡器放行", "I进支线按钮"] ("I0说明")
            (unwired) string[] ["I出支线按钮", "I主线顶升按钮", "I主线下降按钮", "I支线顶升按钮", "I支线下降按钮", "I气压报警", "未使用", "未使用"] ("I0说明")
            n735 = local read "间隙位移(mm)"() -> (w1264:dbl)
            n736 = Greater Or Equal?(x=w1264, y=4.0) -> (x >= y?=w1262:bool)
            n737 = case shown="真" w1262 {
              frame False {
              }
              frame True {
                n738 = local write "测头机构轴使能"(FALSE ("测头机构轴使能")) -> ()
              }
            }
          }
          frame #2 {
            (unwired) string[] ["I电动缸SRDY", "I电动缸ZSPD", "I电动缸ALRM", "I间隙进给SRDY", "I间隙进给ZSPD", "I间隙进给ALRM", "I间隙旋转SRPD", "I间隙旋转ZSPD"] ("I0说明")
            n739 = local read "测头机构轴位置(mm)"() -> (w1268:dbl)
            n740 = Greater Or Equal?(x=w1268, y=90.0) -> (x >= y?=w1266:bool)
            n741 = case shown="假" w1266 {
              frame False {
                w1269 = T5."Enabled" ("禁用")
                n742 = property on="测头气缸右移" class="Bool"("DisabledEnum"=w1269) -> ()  [unwired: 2 in, 2 out]
                n743 = property on="测头气缸左移" class="Bool"("DisabledEnum"=w1269) -> ()  [unwired: 2 in, 2 out]
                n744 = property on="测头气缸右移" class="Bool (严格)"("DisabledEnum"=w1269) -> ()  [unwired: 2 in, 2 out]
                n745 = property on="测头气缸左移" class="Bool (严格)"("DisabledEnum"=w1269) -> ()  [unwired: 2 in, 2 out]
              }
              frame True {
                w1270 = T5."Disabled" ("禁用")
                w1271 = FALSE ("测头气缸右移")
                n746 = local write "测头气缸右移"(w1271) -> ()
                n747 = local write "测头气缸左移"(w1271) -> ()
                n748 = property on="测头气缸右移" class="Bool"("DisabledEnum"=w1270) -> ()  [unwired: 2 in, 2 out]
                n749 = property on="测头气缸左移" class="Bool"("DisabledEnum"=w1270) -> ()  [unwired: 2 in, 2 out]
                n750 = property on="测头气缸右移" class="Bool (严格)"("DisabledEnum"=w1270) -> ()  [unwired: 2 in, 2 out]
                n751 = property on="测头气缸左移" class="Bool (严格)"("DisabledEnum"=w1270) -> ()  [unwired: 2 in, 2 out]
              }
            }
          }
          frame #3 {
            (unwired) string[] ["I间隙旋转ALRM", "I扭矩旋转SRPD", "I扭矩旋转ZSPD", "I扭矩旋转ALRM", "I拧紧机合格", "I拧紧机不合格", "I拧紧机报警", "未使用"] ("I0说明")
          }
        }
      }
      frame #2 {
        n752 = flat-sequence {
          frame #0 {
            (unwired) string[] ["I自制气缸进位", "I自制气缸原位", "I上工位检测", "I本工位检测", "I下工位检测", "I主线顶升上位", "I主线顶升下位", "I支线顶升上位"] ("I0说明")
          }
          frame #1 {
            (unwired) string[] ["I支线顶升下位", "I支线进到位", "I支线退到位", "I位移气缸原位", "I位移气缸进位", "I拧紧机在位", "I电动缸原位", "I电动缸进位"] ("I0说明")
          }
          frame #2 {
            (unwired) string[] ["未使用", "未使用", "未使用", "未使用", "未使用", "未使用", "未使用", "未使用"] ("I0说明")
          }
          frame #3 {
            (unwired) string[] ["未使用", "未使用", "未使用", "未使用", "未使用", "未使用", "未使用", "未使用"] ("I0说明")
          }
        }
        n753 = local read "本测试状态"() -> (w1273:bool)
        n754 = local read "本自动状态"() -> (w1274:bool)
        n755 = local read "本备料状态"() -> (w1272:bool)
        n756 = local write "本测试状态H"(w1273) -> ()
        n757 = local write "本自动状态H"(w1274) -> ()
        n758 = local write "本备料状态H"(w1272) -> ()
      }
      frame #3 {
        n759 = local read "报警工步号"() -> (w1276:dbl)
        n760 = local read "工步号"() -> (w1278:u32)
        n761 = case shown="50" w1278 {
          tunnel: [w1288 "请取胶瓶" ("工步描述") "请对锁紧螺母加力" ("工步描述") "灵敏度测试中" ("工步描述") "有油刚度测试中" ("工步描述") "安装好锁紧螺母后，按顶升按钮，夹具夹紧" ("工步描述") "请点击启动按钮进行试验" ("工步描述") "探头气缸右移" ("工步描述") "电动缸前进找中" ("工步描述") "探头前进测试开始" ("工步描述") "探头退回" ("工步描述") "轴向力测试中" ("工步描述") "测头后退夹抓松开" ("工步描述") "伺服回零" ("工步描述") "力特性试验完成" ("工步描述") "套好输出轴把手，按启动按钮，做回正力试验" ("工步描述") "回正力试验中" ("工步描述") "试验完成，将把手拉回，取下油管，按顶升按钮" ("工步描述") "拆下锁紧螺母和输入轴万向节，按顶升按钮" ("工步描述")] -> w1277
          frame 0, Default {
            n762 = local read "联线按钮"() -> (w1287:bool)
            n763 = case shown="真" w1287 {
              tunnel: ["等待工件" ("工步描述") "等待扫描条码" ("工步描述")] -> w1288
              frame False {
              }
              frame True {
              }
            }
          }
          frame 1 {
          }
          frame 2 {
          }
          frame 3 {
          }
          frame 4 {
          }
          frame 5 {
          }
          frame 6 {
          }
          frame 10 {
          }
          frame 15 {
          }
          frame 20 {
          }
          frame 30 {
          }
          frame 40 {
          }
          frame 45 {
          }
          frame 50 {
          }
          frame 55 {
          }
          frame 60 {
          }
          frame 70 {
          }
          frame 80 {
          }
          frame 56 {
          }
        }
        "工步提示" <- w1277
        n764 = case shown="3" w1276 {
          tunnel: [_ "操作步骤错请取胶瓶" "操作步骤错误请点标" "测头气缸不在原位" "急停被按下" "气压报警" "电动缸伺服报警" "旋转伺服服报警" "测头伺服服报警"] -> w1275
          frame 0, Default {
          }
          frame 1 {
          }
          frame 3 {
          }
          frame 2 {
          }
          frame 4 {
          }
          frame 5 {
          }
          frame 6 {
          }
          frame 7 {
          }
          frame 8 {
          }
        }
        "报警提示" <- w1275
      }
      frame #4 {
        n765 = local read "急停"() -> (w1309:bool)
        n766 = local read "红灯"() -> (w1311:bool)
        n767 = local read "复位"() -> (w1312:bool)
        n768 = local read "复位"() -> (w1314:bool)
        n769 = local read "红灯"() -> (w1313:bool)
        n770 = case shown="假" w1309 {
          frame False {
            w1317 = TRUE ("红灯")
            n771 = local write "红灯"(w1317) -> ()
            n772 = local write "复位"(w1317) -> ()
          }
          frame True {
            w1318 = FALSE ("复位")
            n773 = local write "红灯"(w1318) -> ()
            n774 = local write "复位"(w1318) -> ()
          }
        }
        n775 = Or(x=w1311, y=w1312) -> (x .or. y?=w1310:bool)
        n776 = case shown="真" w1310 {
          frame False {
          }
          frame True {
            n777 = local write "回零完成"(FALSE ("夹头夹紧控制")) -> ()
          }
        }
        n778 = local read "停止"() -> (w1316:bool)
        n779 = Compound Arithmetic op=OR(w1314, w1316, w1313) -> (w1315:bool)
        n780 = case shown="真" w1315 {
          frame False {
          }
          frame True {
            n781 = local read "测头机构电机"() -> (w1320:u32)
            n782 = local read "旋转齿条电机"() -> (w1321:u32)
            n783 = local read "电动缸电机"() -> (w1322:u32)
            n784 = call "PCI1220U停止.vi"("AxisHandle IN"=w1321) -> ()  [unwired: 9 in, 2 out]
            n785 = call "PCI1220U停止.vi"("AxisHandle IN"=w1322) -> ()  [unwired: 9 in, 2 out]
            n786 = call "PCI1220U停止.vi"("AxisHandle IN"=w1320) -> ()  [unwired: 9 in, 2 out]
          }
        }
      }
      frame #5 {
        n787 = local read "齿条扭矩(Nm)"() -> (w1325:dbl)
        n788 = local read "黄灯"() -> (w1323:bool)
        n789 = local read "旋转齿条轴左转"() -> (w1331:bool)
        n790 = Absolute Value(x=w1325) -> (abs(x)=w1330:dbl)
        n791 = local read "旋转齿条轴右转"() -> (w1326:bool)
        n792 = Not(x=w1331) -> (.not. x?=w1327:bool)
        n793 = Less?(x=w1330, y=20.0) -> (x < y?=w1328:bool)
        n794 = Compound Arithmetic op=AND(w1326, w1327, w1328, w1323) -> (w1324:bool)
        n795 = case shown="真" w1324 {
          frame False {
          }
          frame True {
            n796 = flat-sequence {
              tunnel: [w1335] -> w1333
              tunnel: w1333 -> [w1337]
              tunnel: [w1337] -> w1332
              tunnel: w1332 -> [w1348]
              frame #0 {
                n797 = local read "旋转齿条电机"() -> (w1334:u32)
                n798 = call "PCI1220U运行.vi"("方向"=enum32{"Negative", "Positive"}."Negative" ("Direction"), "AxisHandle IN"=w1334) -> ("AxisHandle OUT"=w1335:u32)  [unwired: 9 in]
              }
              frame #1 {
                n799 = while {
                  stop <- w1341 stop-if-true
                  n800 = Wait (ms)(milliseconds to wait=u32 50 ("毫秒倍数")) -> ()  [unwired: 1 out]
                  n801 = local read "齿条扭矩(Nm)"() -> (w1346:dbl)
                  n802 = local read "旋转齿条轴右转"() -> (w1343:bool)
                  n803 = local read "红灯"() -> (w1338:bool)
                  n804 = local read "复位"() -> (w1339:bool)
                  n805 = Absolute Value(x=w1346) -> (abs(x)=w1345:dbl)
                  n806 = Not(x=w1343) -> (.not. x?=w1340:bool)
                  n807 = Greater?(x=w1345, y=10.0) -> (0:w1342:bool)
                  n808 = Compound Arithmetic op=OR(w1342, w1340, w1339, w1338) -> (w1341:bool)
                }
              }
              frame #2 {
                n809 = call "PCI1220U停止.vi"("AxisHandle IN"=w1348) -> ()  [unwired: 9 in, 2 out]
              }
            }
          }
        }
      }
      frame #6 {
        n810 = local read "齿条扭矩(Nm)"() -> (w1353:dbl)
        n811 = local read "旋转齿条轴右转"() -> (w1357:bool)
        n812 = Absolute Value(x=w1353) -> (abs(x)=w1352:dbl)
        n813 = local read "旋转齿条轴左转"() -> (w1355:bool)
        n814 = local read "黄灯"() -> (w1349:bool)
        n815 = Not(x=w1357) -> (.not. x?=w1354:bool)
        n816 = Less?(x=w1352, y=20.0) -> (x < y?=w1350:bool)
        n817 = Compound Arithmetic op=AND(w1355, w1354, w1350, w1349) -> (w1356:bool)
        n818 = case shown="真" w1356 {
          frame False {
          }
          frame True {
            n819 = flat-sequence {
              tunnel: [w1361] -> w1359
              tunnel: w1359 -> [w1363]
              tunnel: [w1363] -> w1358
              tunnel: w1358 -> [w1374]
              frame #0 {
                n820 = local read "旋转齿条电机"() -> (w1360:u32)
                n821 = call "PCI1220U运行.vi"("方向"=enum32{"Negative", "Positive"}."Positive" ("Direction"), "AxisHandle IN"=w1360) -> ("AxisHandle OUT"=w1361:u32)  [unwired: 9 in]
              }
              frame #1 {
                n822 = while {
                  stop <- w1366 stop-if-true
                  n823 = Wait (ms)(milliseconds to wait=u32 50 ("毫秒倍数")) -> ()  [unwired: 1 out]
                  n824 = local read "齿条扭矩(Nm)"() -> (w1372:dbl)
                  n825 = local read "旋转齿条轴左转"() -> (w1369:bool)
                  n826 = local read "红灯"() -> (w1364:bool)
                  n827 = local read "复位"() -> (w1365:bool)
                  n828 = Absolute Value(x=w1372) -> (abs(x)=w1371:dbl)
                  n829 = Not(x=w1369) -> (.not. x?=w1367:bool)
                  n830 = Greater?(x=w1371, y=10.0) -> (0:w1368:bool)
                  n831 = Compound Arithmetic op=OR(w1365, w1364, w1368, w1367) -> (w1366:bool)
                }
              }
              frame #2 {
                n832 = call "PCI1220U停止.vi"("AxisHandle IN"=w1374) -> ()  [unwired: 9 in, 2 out]
              }
            }
          }
        }
      }
      frame #7 {
        n833 = local read "齿条推拉力(N)"() -> (w1379:dbl)
        n834 = local read "电动缸前进"() -> (w1376:bool)
        n835 = local read "电动缸后退"() -> (w1375:bool)
        n836 = Absolute Value(x=w1379) -> (abs(x)=w1383:dbl)
        n837 = local read "黄灯"() -> (w1377:bool)
        n838 = Not(x=w1375) -> (.not. x?=w1380:bool)
        n839 = Less?(x=w1383, y=1000.0) -> (x < y?=w1381:bool)
        n840 = Compound Arithmetic op=AND(w1376, w1380, w1377, w1381) -> (w1378:bool)
        n841 = case shown="真" w1378 {
          frame False {
          }
          frame True {
            n842 = flat-sequence {
              tunnel: [w1387] -> w1385
              tunnel: w1385 -> [w1389]
              tunnel: [w1389] -> w1384
              tunnel: w1384 -> [w1400]
              frame #0 {
                n843 = local read "电动缸电机"() -> (w1386:u32)
                n844 = call "PCI1220U运行.vi"("方向"=enum32{"Negative", "Positive"}."Positive" ("Direction"), "AxisHandle IN"=w1386) -> ("AxisHandle OUT"=w1387:u32)  [unwired: 9 in]
              }
              frame #1 {
                n845 = while {
                  stop <- w1397 stop-if-true
                  n846 = local read "电动缸前进"() -> (w1394:bool)
                  n847 = local read "齿条推拉力(N)"() -> (w1391:dbl)
                  n848 = Wait (ms)(milliseconds to wait=u32 50 ("毫秒倍数")) -> ()  [unwired: 1 out]
                  n849 = Absolute Value(x=w1391) -> (abs(x)=w1393:dbl)
                  n850 = local read "红灯"() -> (w1395:bool)
                  n851 = local read "复位"() -> (w1396:bool)
                  n852 = Greater?(x=w1393, y=1000.0) -> (0:w1390:bool)
                  n853 = Not(x=w1394) -> (.not. x?=w1398:bool)
                  n854 = Compound Arithmetic op=OR(w1396, w1395, w1398, w1390) -> (w1397:bool)
                }
              }
              frame #2 {
                n855 = call "PCI1220U停止.vi"("AxisHandle IN"=w1400) -> ()  [unwired: 9 in, 2 out]
              }
            }
          }
        }
      }
      frame #8 {
        n856 = local read "电动缸前进"() -> (w1401:bool)
        n857 = local read "齿条推拉力(N)"() -> (w1405:dbl)
        n858 = local read "电动缸后退"() -> (w1402:bool)
        n859 = Absolute Value(x=w1405) -> (abs(x)=w1409:dbl)
        n860 = local read "黄灯"() -> (w1403:bool)
        n861 = Not(x=w1401) -> (.not. x?=w1406:bool)
        n862 = Less?(x=w1409, y=1000.0) -> (x < y?=w1407:bool)
        n863 = Compound Arithmetic op=AND(w1402, w1406, w1403, w1407) -> (w1404:bool)
        n864 = case shown="真" w1404 {
          frame False {
          }
          frame True {
            n865 = flat-sequence {
              tunnel: [w1413] -> w1411
              tunnel: w1411 -> [w1415]
              tunnel: [w1415] -> w1410
              tunnel: w1410 -> [w1426]
              frame #0 {
                n866 = local read "电动缸电机"() -> (w1412:u32)
                n867 = call "PCI1220U运行.vi"("方向"=enum32{"Negative", "Positive"}."Negative" ("Direction"), "AxisHandle IN"=w1412) -> ("AxisHandle OUT"=w1413:u32)  [unwired: 9 in]
              }
              frame #1 {
                n868 = while {
                  stop <- w1423 stop-if-true
                  n869 = local read "电动缸后退"() -> (w1420:bool)
                  n870 = local read "齿条推拉力(N)"() -> (w1419:dbl)
                  n871 = Wait (ms)(milliseconds to wait=u32 50 ("毫秒倍数")) -> ()  [unwired: 1 out]
                  n872 = Absolute Value(x=w1419) -> (abs(x)=w1417:dbl)
                  n873 = local read "红灯"() -> (w1422:bool)
                  n874 = local read "复位"() -> (w1421:bool)
                  n875 = Greater?(x=w1417, y=1000.0) -> (0:w1416:bool)
                  n876 = Not(x=w1420) -> (.not. x?=w1424:bool)
                  n877 = Compound Arithmetic op=OR(w1421, w1422, w1424, w1416) -> (w1423:bool)
                }
              }
              frame #2 {
                n878 = call "PCI1220U停止.vi"("AxisHandle IN"=w1426) -> ()  [unwired: 9 in, 2 out]
              }
            }
          }
        }
      }
      frame #9 {
        n879 = local read "测头机构轴后退"() -> (w1427:bool)
        n880 = local read "测头机构轴前进"() -> (w1428:bool)
        n881 = local read "黄灯"() -> (w1429:bool)
        n882 = Not(x=w1427) -> (.not. x?=w1431:bool)
        n883 = Compound Arithmetic op=AND(w1428, w1431, w1429) -> (w1430:bool)
        n884 = case shown="真" w1430 {
          frame False {
          }
          frame True {
            n885 = flat-sequence {
              tunnel: [w1435] -> w1433
              tunnel: w1433 -> [w1437]
              tunnel: [w1437] -> w1432
              tunnel: w1432 -> [w1444]
              frame #0 {
                n886 = local read "测头机构电机"() -> (w1434:u32)
                n887 = call "PCI1220U运行.vi"("方向"=enum32{"Negative", "Positive"}."Positive" ("Direction"), "AxisHandle IN"=w1434) -> ("AxisHandle OUT"=w1435:u32)  [unwired: 9 in]
              }
              frame #1 {
                n888 = while {
                  stop <- w1441 stop-if-true
                  n889 = local read "测头机构轴前进"() -> (w1438:bool)
                  n890 = Wait (ms)(milliseconds to wait=u32 50 ("毫秒倍数")) -> ()  [unwired: 1 out]
                  n891 = local read "红灯"() -> (w1439:bool)
                  n892 = local read "复位"() -> (w1440:bool)
                  n893 = Not(x=w1438) -> (.not. x?=w1442:bool)
                  n894 = Compound Arithmetic op=OR(w1440, w1439, w1442) -> (w1441:bool)
                }
              }
              frame #2 {
                n895 = call "PCI1220U停止.vi"("AxisHandle IN"=w1444) -> ()  [unwired: 9 in, 2 out]
              }
            }
          }
        }
      }
      frame #10 {
        n896 = local read "测头机构轴前进"() -> (w1445:bool)
        n897 = local read "测头机构轴后退"() -> (w1446:bool)
        n898 = local read "黄灯"() -> (w1447:bool)
        n899 = Not(x=w1445) -> (.not. x?=w1449:bool)
        n900 = Compound Arithmetic op=AND(w1446, w1449, w1447) -> (w1448:bool)
        n901 = case shown="真" w1448 {
          frame False {
          }
          frame True {
            n902 = flat-sequence {
              tunnel: [w1453] -> w1451
              tunnel: w1451 -> [w1455]
              tunnel: [w1455] -> w1450
              tunnel: w1450 -> [w1462]
              frame #0 {
                n903 = local read "测头机构电机"() -> (w1452:u32)
                n904 = call "PCI1220U运行.vi"("方向"=enum32{"Negative", "Positive"}."Negative" ("Direction"), "AxisHandle IN"=w1452) -> ("AxisHandle OUT"=w1453:u32)  [unwired: 9 in]
              }
              frame #1 {
                n905 = while {
                  stop <- w1459 stop-if-true
                  n906 = local read "测头机构轴后退"() -> (w1456:bool)
                  n907 = Wait (ms)(milliseconds to wait=u32 50 ("毫秒倍数")) -> ()  [unwired: 1 out]
                  n908 = local read "红灯"() -> (w1458:bool)
                  n909 = local read "复位"() -> (w1457:bool)
                  n910 = Not(x=w1456) -> (.not. x?=w1460:bool)
                  n911 = Compound Arithmetic op=OR(w1457, w1458, w1460) -> (w1459:bool)
                }
              }
              frame #2 {
                n912 = call "PCI1220U停止.vi"("AxisHandle IN"=w1462) -> ()  [unwired: 9 in, 2 out]
              }
            }
          }
        }
      }
    }
    n913 = Wait (ms)(milliseconds to wait=u32 50 ("毫秒倍数")) -> ()  [unwired: 1 out]
    n914 = local read "停止"() -> (w1253:bool)
  }
  n915 = flat-sequence {
    tunnel: [w1466] -> w2
    tunnel: [w1464] -> w1
    tunnel: w2 -> [w1476]
    tunnel: w1 -> [w1475]
    frame #0 {
      n916 = First Call?() -> (First Call?: T/F=w1463:bool)
      n917 = case shown="真" w1463 {
        frame False {
        }
        frame True {
          n918 = while {
            i -> [w1471]
            stop <- w1469 stop-if-true
            w1474 = TRUE ("电动缸使能")
            n919 = local write "回零完成"(FALSE ("回零完成")) -> ()
            n920 = local write "测头机构轴使能"(w1474) -> ()
            n921 = local write "旋转齿条轴使能"(w1474) -> ()
            n922 = local write "电动缸使能"(w1474) -> ()
            n923 = Wait Until Next ms Multiple(millisecond multiple=u32 50 ("毫秒倍数")) -> ()  [unwired: 1 out]
            n924 = Greater Or Equal?(x=w1471, y=30) -> (x >= y?=w1469:bool)
          }
        }
      }
      n925 = call "ADO Connection Create.vi"() -> ("error out"=w1467:errorcluster, "ADODB._Connection Out"=w1468:refnum<k7>)  [unwired: 10 in]
      n926 = call "ADO Connection Open.vi"("error in (no error)"=w1467, "ConnectionString"="Provider=Microsoft.Jet.OLEDB.4.0;Data Source=D:\\Q14070-Z060人机界面\\参数\\参数Z060.mdb;Persist Security Info=False;Jet OLEDB:Database Password=123;", "ADODB._Connection In"=w1468) -> ("error out"=w1464:errorcluster, "ADODB._Connection Out"=w1466:refnum<k7>)  [unwired: 7 in]
    }
    frame #1 {
      n927 = while {
        tunnel: w1476 -> [w1478]
        tunnel: w1475 -> [w1477]
        stop <- w1482 stop-if-true
        n928 = Wait (ms)(milliseconds to wait=u32 50 ("等待时间（毫秒）")) -> ()  [unwired: 1 out]
        n929 = First Call?() -> (First Call?: T/F=w1481:bool)
        n930 = Or(x=w1481, y="参数加载") -> (x .or. y?=w1480:bool)
        n931 = case shown="真" w1480 {
          tunnel: w1478 -> [_ w1485]
          tunnel: w1477 -> [_ w1484]
          frame False {
          }
          frame True {
            n932 = stacked-sequence {
              tunnel: w1485 -> [w1491 w1502 w1558]
              tunnel: w1484 -> [w1486 _ _]
              frame #0 {
                n933 = call "SQL Execute.vi"("error in (no error)"=w1486, "Command Text"="SELECT * FROM 测试参数表", "ADODB._Connection In"=w1491) -> ("Data"=w1489:string[][])  [unwired: 5 in, 3 out]
                n934 = Index Array(array=w1489, index (col)=0 ("索引 (行)")) -> (element=w1493:string[])  [unwired: 1 in]
                n935 = Array Size(array=w1493) -> (size(s)=w1488:i32)
                "型号数量" <- w1488
                n936 = while {
                  shift-right: [w1500] -> w1492
                  shift-left: i32[] [] -> [w1499]
                  tunnel: w1488 -> [w1497]
                  i -> [w1498]
                  stop <- w1496 stop-if-true
                  n937 = Greater Or Equal?(x=w1498, y=w1497) -> (x >= y?=w1496:bool)
                  n938 = Build Array (concatenate)(w1499, w1498) -> (w1500:i32[])
                }
                n939 = Build Cluster Array "索引与捆绑簇数组"(w1493, w1492) -> (w1487:cluster{"String":string, i32}[])
                n940 = property on="型号选择" class="Ring (严格)"("StringsAndValues[]"=w1487) -> ()  [unwired: 2 in, 2 out]
              }
              frame #1 {
                n941 = property on="型号选择" class="Ring (严格)"() -> ("RingText.Text"=w1503:string)  [unwired: 2 in, 2 out]
                n942 = call "创建文本2"("型号选择"=w1503) -> ("Result"=w1507:string)  [unwired: 13 in, 1 out]
                n943 = call "SQL Execute.vi"("Command Text"=w1507, "ADODB._Connection In"=w1502) -> ("Data"=w1506:string[][])  [unwired: 6 in, 3 out]
                n944 = Index Array(array=w1506, index (row)=0 ("索引 (行)")) -> (element=w1504:string[])  [unwired: 1 in]
                n945 = Fract/Exp String To Number ("分数/指数字符串至数值转换")(string=w1504) -> (number=w1501:dbl[])  [unwired: 3 in, 1 out]
                n946 = stacked-sequence {
                  tunnel: w1501 -> [w1534]
                  frame #0 {
                    n947 = Index Array ("索引数组")(array=w1534, index #1=2 ("索引"), index #2=3 ("索引"), index #3=4 ("索引"), index #4=5 ("索引"), index #5=6 ("索引"), index #6=7 ("索引"), index #7=8 ("索引"), index #8=9 ("索引"), index #9=10 ("索引"), index #10=11 ("索引"), index #11=12 ("索引"), index #12=13 ("索引"), index #13=14 ("索引"), index #14=15 ("索引"), index #15=16 ("索引"), index #16=17 ("索引"), index #17=18 ("索引"), index #18=19 ("索引")) -> (element #1=w1533:dbl, element #2=w1532:dbl, element #3=w1531:dbl, element #4=w1530:dbl, element #5=w1529:dbl, element #6=w1528:dbl, element #7=w1527:dbl, element #8=w1526:dbl, element #9=w1525:dbl, element #10=w1524:dbl, element #11=w1517:dbl, element #12=w1516:dbl, element #13=w1515:dbl, element #14=w1514:dbl, element #15=w1513:dbl, element #16=w1512:dbl, element #17=w1509:dbl, element #18=w1508:dbl)
                    n948 = local write "测头机构轴移动速度"(w1533) -> ()
                    n949 = local write "总圈数标准"(w1509) -> ()
                    n950 = local write "总圈数最大值"(w1508) -> ()
                    n951 = local write "平均轴向力标准(N) max"(w1512) -> ()
                    n952 = local write "平均轴向力标准(N)"(w1513) -> ()
                    n953 = local write "测头机构轴检测位"(w1532) -> ()
                    n954 = local write "测头机构轴后退位"(w1530) -> ()
                    n955 = local write "测头机构轴待检位"(w1531) -> ()
                    n956 = local write "旋转齿条轴找帽转速"(w1526) -> ()
                    n957 = local write "旋转齿条轴测量转速"(w1525) -> ()
                    n958 = local write "总行程标准(mm)"(w1517) -> ()
                    n959 = local write "最大轴向力标准(N)"(w1515) -> ()
                    n960 = local write "齿条移动速度"(w1529) -> ()
                    n961 = local write "齿条左极限"(w1528) -> ()
                    n962 = local write "齿条右极限"(w1527) -> ()
                    n963 = local write "力波动标准(N)"(w1514) -> ()
                    n964 = local write "总行程最大值"(w1516) -> ()
                    n965 = local write "测量点扭矩"(w1524) -> ()
                  }
                }
              }
              frame #2 {
                n966 = call "SQL Execute.vi"("Command Text"="SELECT * FROM 传感器校验表 where ID='1'", "ADODB._Connection In"=w1558) -> ("Data"=w1560:string[][])  [unwired: 6 in, 3 out]
                n967 = Index Array(array=w1560) -> (element=w1561:string[])  [unwired: 2 in]
                n968 = Fract/Exp String To Number ("分数/指数字符串至数值转换")(string=w1561) -> (number=w1551:dbl[])  [unwired: 3 in, 1 out]
                n969 = Index Array(array=w1551, index #1=1 ("索引"), index #2=2 ("索引"), index #3=3 ("索引"), index #4=4 ("索引"), index #5=5 ("索引"), index #6=6 ("索引")) -> (element #1=w1550:dbl, element #2=w1549:dbl, element #3=w1548:dbl, element #4=w1547:dbl, element #5=w1546:dbl, element #6=w1545:dbl)
                n970 = local write "间隙位移零点偏移"(w1550) -> ()
                n971 = local write "间隙位移比例偏移"(w1549) -> ()
                n972 = local write "齿条推拉力零点偏移"(w1548) -> ()
                n973 = local write "齿条推拉力比例偏移"(w1547) -> ()
                n974 = local write "齿条扭矩零点偏移"(w1546) -> ()
                n975 = local write "齿条扭矩比例偏移"(w1545) -> ()
              }
            }
          }
        }
        n976 = local read "停止"() -> (w1482:bool)
        "ADODB._Connection Out 2" <- w1478
      }
    }
  }
  n977 = while {
    stop <- w1563 stop-if-true
    n978 = local read "rfid工步号"() -> (w1562:u32)
    n979 = case shown="10" w1562 {
      frame 0, Default {
      }
      frame 10 {
        n980 = flat-sequence {
          tunnel: [w1573] -> w1567
          tunnel: w1567 -> [w1575]
          tunnel: [w1574] -> w1566
          tunnel: w1566 -> [w1577]
          tunnel: [w1577] -> w1565
          tunnel: w1565 -> [w1580]
          frame #0 {
            n981 = while {
              stop <- w1568 stop-if-true
              n982 = local read "rfid触发"() -> (w1568:bool)
              n983 = Wait Until Next ms Multiple(millisecond multiple=u32 50 ("毫秒倍数")) -> ()  [unwired: 1 out]
            }
          }
          frame #1 {
            n984 = local write "芯片ID"("" ("随行板ID")) -> ()
            n985 = local write "rfid完成"(FALSE ("RFID完成")) -> ()
            n986 = local write "rfid触发"(FALSE ("RFID读取触发")) -> ()
          }
          frame #2 {
            n987 = local read "Z060BRFID"() -> (w1573:string)
            n988 = local write "芯片ID"(w1573) -> ()
          }
          frame #3 {
            n989 = call "查询产品ID.vi"("芯片编码"=w1575) -> ("产品ID"=w1574:string)  [unwired: 8 in, 2 out]
            "读取产品ID" <- w1574
          }
          frame #4 {
            n990 = Wait (ms)(milliseconds to wait=u32 500 ("等待时间（毫秒）")) -> ()  [unwired: 1 out]
          }
          frame #5 {
            n991 = call "查询上序合格.vi"("产品ID"=w1580) -> ("本序已做"=w1578:bool, "上序合格"=w1579:bool)  [unwired: 8 in, 1 out]
            n992 = Not(x=w1579) -> (.not. x?=w1581:bool)
            n993 = local write "上序合格"(w1579) -> ()
            n994 = local write "本序已做"(w1578) -> ()
            n995 = local write "上序不合格"(w1581) -> ()
          }
          frame #6 {
            n996 = local write "rfid完成"(TRUE ("RFID读取完成")) -> ()
            n997 = Wait Until Next ms Multiple(millisecond multiple=u32 500 ("毫秒倍数")) -> ()  [unwired: 1 out]
          }
          frame #7 {
            "rfid工步号" <- 15.0 ("工步号")
          }
        }
      }
      frame 210 {
        n998 = local read "读取产品ID"() -> (w1585:string)
        n999 = local write "产品ID"(w1585) -> ()
      }
    }
    n1000 = Wait Until Next ms Multiple(millisecond multiple=u32 50 ("毫秒倍数")) -> ()  [unwired: 1 out]
    n1001 = local read "停止"() -> (w1563:bool)
  }
  n1002 = flat-sequence {
    tunnel: [w1586] -> w4
    tunnel: w4 -> [w1592]
    tunnel: [w1591] -> w3
    tunnel: w3 -> [w1658]
    frame #0 {
      n1003 = call "PCI1240U初始化.vi"() -> ("旋转电机"=→"旋转齿条电机":u32, "电动缸电机"=→"电动缸电机":u32, "DeviceHandle"=→"DeviceHandle":u32, "进给电机"=→"测头机构电机":u32)  [unwired: 6 in, 2 out]
      n1004 = call "PCI8622配置.vi"() -> ("DeviceID"=w1586:i32)  [unwired: 11 in]
    }
    frame #1 {
      n1005 = while {
        tunnel: w1592 -> [w1594]
        tunnel: [w1593] -> w1591
        stop <- "停止" stop-if-true
        n1006 = stacked-sequence {
          tunnel: w1594 -> [_ _ w1634]
          tunnel: [_ _ w1634] -> w1593
          frame #0 {
            n1007 = local read "测头机构电机"() -> (w1603:u32)
            n1008 = Boolean To (0,1)(Boolean="测头机构轴使能") -> (0, 1=w1601:i16)
            n1009 = call <userlib>:"Acm_AxSetSvOn.vi"("OnOff"=w1601, "AxisHandle"=w1603) -> ("AxisHandle"=w1600:u32)  [unwired: 1 in, 2 out]
            n1010 = call "PCI1220U进给轴速度设置.vi"("Change Velocity"="测头机构轴速度(mm/s)", "AxisHandle IN"=w1600) -> ("AxisHandle OUT"=w1598:u32)  [unwired: 9 in]
            n1011 = call "PCI1220U进给轴读取位置.vi"("AxisHandle IN"=w1598) -> ("位置"=→"测头机构轴位置(mm)":dbl)  [unwired: 9 in, 1 out]
          }
          frame #1 {
            n1012 = local read "电动缸电机"() -> (w1613:u32)
            n1013 = local read "旋转齿条电机"() -> (w1612:u32)
            n1014 = Boolean To (0,1)(Boolean="电动缸使能") -> (0, 1=w1617:i16)
            n1015 = Boolean To (0,1)(Boolean="旋转齿条轴使能") -> (0, 1=w1611:i16)
            n1016 = call <userlib>:"Acm_AxSetSvOn.vi"("OnOff"=w1611, "AxisHandle"=w1612) -> ("AxisHandle"=w1614:u32)  [unwired: 1 in, 2 out]
            n1017 = call <userlib>:"Acm_AxSetSvOn.vi"("OnOff"=w1617, "AxisHandle"=w1613) -> ("AxisHandle"=w1616:u32)  [unwired: 1 in, 2 out]
            n1018 = call "PCI1220U扭矩轴速度设置.vi"("Change Velocity"="旋转齿条轴速度(°/s)", "AxisHandle IN"=w1614) -> ("AxisHandle OUT"=w1615:u32)  [unwired: 9 in]
            n1019 = call "PCI1240电动缸速度设置.vi"("Change Velocity"="电动缸速度(mm/s)", "AxisHandle IN"=w1616) -> ("AxisHandle OUT"=w1604:u32)  [unwired: 9 in]
            n1020 = call "PCI1220U扭矩轴读取位置.vi"("AxisHandle IN"=w1615) -> ("位置"=→"旋转齿条轴位置(°)":dbl)  [unwired: 9 in, 1 out]
            n1021 = call "PCI1240电动缸读取位置.vi"("AxisHandle IN"=w1604) -> ("位置"=→"电动缸位置(mm)":dbl)  [unwired: 9 in, 1 out]
          }
          frame #2 {
            w1650 = 0  # nRetSizeWords
            w1651 = 2048  # nReadSizeWords
            # "hDevice"
            n1022 = Initialize Array(u16 0, 2048 ("dimension size")) -> (w1641:u16[])
            n1023 = dll-call lib="PCI8622_32.dll" fn="PCI8622_ReadDeviceProAD_Npt" label="ReadDeviceProAD_Npt"("hDevice"=w1634, "ADBuffer[]"=w1641, "nReadSizeWords"=w1651, "nRetSizeWords"=w1650) -> ("ADBuffer[]"=w1644:u16[])  [unwired: 7 in, 2 out]
            n1024 = Divide(x=w1644, y=65536.01) -> (x/y=w1645:dbl[])
            n1025 = Multiply(x=w1645, y=20) -> (x*y=w1648:dbl[])
            n1026 = Subtract(x=w1648, y=10) -> (x-y=w1640:dbl[])
            n1027 = Decimate 1D Array ("抽取一维数组")(w1640) -> (w1628:dbl[], w1629:dbl[], w1627:dbl[])  [unwired: 5 out]
            n1028 = Add Array Elements(numeric array=w1628) -> (sum=w1637:dbl)
            n1029 = Add Array Elements(numeric array=w1627) -> (sum=w1638:dbl)
            n1030 = Array Size(array=w1628) -> (size(s)=w1636:i32)
            n1031 = Add Array Elements(numeric array=w1629) -> (sum=w1633:dbl)
            n1032 = Array Size(array=w1627) -> (size(s)=w1639:i32)
            n1033 = Array Size(array=w1629) -> (size(s)=w1635:i32)
            n1034 = Divide(x=w1637, y=w1636) -> (x/y=w1626:dbl)
            n1035 = Divide(x=w1638, y=w1639) -> (x/y=w1620:dbl)
            n1036 = Divide(x=w1633, y=w1635) -> (x/y=w1623:dbl)
            n1037 = Subtract(x=w1620, y=4.43) -> (x-y=w1618:dbl)
            n1038 = Multiply(x=w1626, y=2.0) -> (x*y=w1621:dbl)
            n1039 = Multiply(x=w1623, y=200.0) -> (x*y=w1622:dbl)
            n1040 = local read "间隙位移比例偏移"() -> (w1655:dbl)
            n1041 = local read "间隙位移零点偏移"() -> (w1654:dbl)
            n1042 = local read "齿条扭矩零点偏移"() -> (w1656:dbl)
            n1043 = local read "齿条扭矩比例偏移"() -> (w1657:dbl)
            n1044 = local read "齿条推拉力比例偏移"() -> (w1653:dbl)
            n1045 = local read "齿条推拉力零点偏移"() -> (w1652:dbl)
            n1046 = call "传感器校订.vi"("零点"=w1656, "比例"=w1657, "传感器"=w1621) -> ("示值"=→"齿条扭矩(Nm)":dbl)  [unwired: 8 in]
            n1047 = call "传感器校订.vi"("零点"=w1654, "比例"=w1655, "传感器"=w1618) -> ("示值"=→"间隙位移(mm)":dbl)  [unwired: 8 in]
            n1048 = call "传感器校订.vi"("零点"=w1652, "比例"=w1653, "传感器"=w1622) -> ("示值"=→"齿条推拉力(N)":dbl)  [unwired: 8 in]
          }
        }
        n1049 = Wait Until Next ms Multiple(millisecond multiple=u32 50 ("毫秒倍数")) -> ()  [unwired: 1 out]
      }
    }
    frame #2 {
      n1050 = dll-call lib="PCI8622_32.dll" fn="PCI8622_StopDeviceProAD" label="StopDeviceProAD"("hDevice"=w1658) -> ("hDevice"=w1659:i32)  [unwired: 4 in, 2 out]
      n1051 = dll-call lib="PCI8622_32.dll" fn="PCI8622_ReleaseDeviceProAD" label="ReleaseDeviceProAD"("hDevice"=w1659) -> ()  [unwired: 5 in, 2 out]
      n1052 = dll-call lib="PCI8622_32.dll" fn="PCI8622_ReleaseDevice" label="ReleaseDevice"("hDevice"=w1658) -> ()  [unwired: 5 in, 2 out]
    }
  }
